vi "!GviewerMain.vi"() -> ()   [LabVIEW 2020, in "Sgraph_lib_V1.lvlib" / "Gviewer.lvclass"]
doc: "Main Graph Viewer.\nSeveral instances of this viewer can run simultaneously."
uses:
  Gviewer.lvclass
  controls/Typedef_Live.ctl
  Gserver/controls/Typedef_Gviewer-Query.ctl
  Gserver/controls/Typedef_QueryType.ctl
  controls/KeyPress.ctl
  <vilib>/event_ctls.llb/eventvkey.ctl
  Gviewer.lvclass/Gviewer.ctl
  FAMM/controls/FAMM_reply_datagram.ctl
  FAMM/controls/FAMM_reply_WAQdata.ctl
  FAMM/controls/FAMM_reply_EAQdata.ctl
  FAMM/controls/FAMM_reply_PAQdata.ctl
  controls/EditTagOneTag.ctl
  controls/Typedef_SelProperties.ctl
  controls/Typedef_LineType.ctl
  controls/Typedef_PresetSave.ctl
  controls/AutoScale.ctl
  controls/ToolBarAppearance.ctl
  controls/Typedef_Gserver-Replies.ctl
  controls/Typedef_ServerActions.ctl
  Common/controls/ToolTypeEnum.ctl
  controls/YgraphDef.ctl
  controls/MinMax.ctl
  Gserver/Gserver.lvclass
  FAMM/FAMM.lvclass
  Builds/Sgraph_lib_V1.lvlib
panel:
  out "TimeSpanText":string
  out "Key UP":T1 {"Time" format="%<%.3X>T"}
  out "Key DN":T1 {"Time" format="%<%.3X>T"}
  in  "StartupTagList":string[](array[string])
  in  "Gserver-Queue":refnum<queue>
  in  "GviewName":string="Gview-01"
  in  "Live":T3
  out "ToolBar":picture
  out "Graph":cluster{dbl[], "data":dbl[]}[](graph)
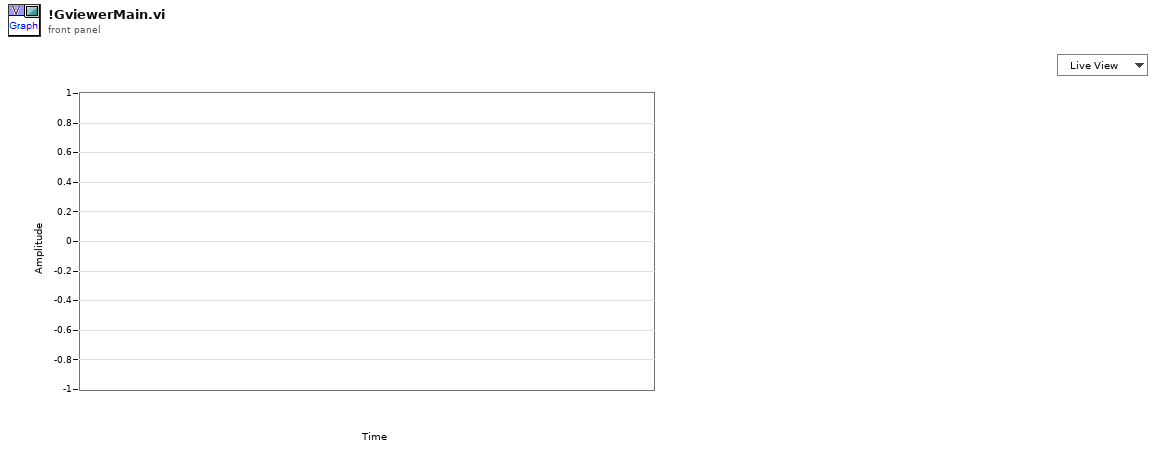
[diagram p1: front panel]
types:
  T1 = typedef "Sgraph_lib_V1.lvlib/Gviewer.lvclass/KeyPress.ctl" = cluster{"Char":i16, "VKey":T2, "Shift":bool, "Ctrl":bool, "Time":timestamp}
  T2 = typedef "eventvkey.ctl" = enum16{"ASCII", "Enter", "Return", "Shift", "Ctrl", "Alt", "Cmd", "Opt", "Caps", "NumLock", "Clear", "Break", "Up", "Down", "Left", "Right", "Insert", "Delete", "Home", "End", "PageUp", "PageDown", "Escape", "Help", "Pause", "ScrollLock", "F1", "F2", "F3", "F4", "F5", "F6", "F7", "F8", "F9", "F10", "F11", "F12", "F13", "F14", "F15", "F16", "F17", "F18", "F19", "F20", "F21", "F22", "F23", "F24", "Play", "VolumeUp", "VolumeDown", "Mute", "Two Byte Char"}
  T3 = typedef "Sgraph_lib_V1.lvlib/Gviewer.lvclass/Typedef_Live.ctl" = enum16{"Live View", "Freeze"}
  T4 = typedef "Sgraph_lib_V1.lvlib/FAMM.lvclass/FAMM_reply_datagram.ctl" = cluster{"GraphName":string, "Time-Start":timestamp, "Time-End":timestamp, "TimeSpan":dbl, "Live":T3, "WAQ_section":T5, "EAQ_section":T6, "PAQ_section":T7, "Layer":i32}
  T5 = typedef "Sgraph_lib_V1.lvlib/FAMM.lvclass/FAMM_reply_WAQdata.ctl" = cluster{"Boolean":bool}
  T6 = typedef "Sgraph_lib_V1.lvlib/FAMM.lvclass/FAMM_reply_EAQdata.ctl" = cluster{"Boolean":bool}
  T7 = typedef "Sgraph_lib_V1.lvlib/FAMM.lvclass/FAMM_reply_PAQdata.ctl" = cluster{"Tags":string[], "time stamp":timestamp[], "DataSection":cluster{"data":dbl[], "max":dbl[], "min":dbl[], "Status":u32[]}[]}
  T8 = typedef "Sgraph_lib_V1.lvlib/Gviewer.lvclass/EditTagOneTag.ctl" = cluster{"TAG":string, "min":dbl, "max":dbl, "Color":u32}
  T9 = typedef "Sgraph_lib_V1.lvlib/Gviewer.lvclass/Typedef_LineType.ctl" = enum16{"num_bare", "num_MinMax_Area", "num_MinMax_Lines", "num_MinMax_Forfor", "num_Max_Area", "num_Max_Line", "num_Max_Forfor", "num_Min_Area", "num_Min_Line", "num_Min_Fosfor", "Boolean_Line_01", "Boolean_Area_01", "Boolean_Fosfor_01", "Boolean_Line_TF", "Boolean_Area_TF", "Boolean_Fosfor_TF", "Boolean_OnOff_Line", "Boolean_OnOff_Area", "Boolean_OnOff_Fosfor", "Boolean_spare", "StringEvent_Line", "StringEvent_TimeLine"}
  T10 = typedef "Sgraph_lib_V1.lvlib/Gviewer.lvclass/Typedef_SelProperties.ctl" = cluster{"Color":u32, "LineType":T9, "max":dbl, "min":dbl}
  T11 = cluster{"EditTagsOpen":bool, "ExitRef":refnum<vi>}
  T12 = typedef "Sgraph_lib_V1.lvlib/Gviewer.lvclass/Typedef_PresetSave.ctl" = cluster{"Save time?":bool, "Presets":T8[], "PresetFilePath":path}
  T13 = typedef "Sgraph_lib_V1.lvlib/Gviewer.lvclass/AutoScale.ctl" = enum16{"FitEqual", "FitMax", "StackEqual", "StackMax", "StackPerType"}
  T14 = typedef "Sgraph_lib_V1.lvlib/Gserver.lvclass/Typedef_QueryType.ctl" = enum16{"Subscribe", "DataRequest", "RequestAllTags", "RequestIniPath", "FAMMstarted", "SetClientOptions", "GviewerUpdate", "OpenNewGraph", "CloseClient", "CloseAllClients", "Close Gserver", "OpenMemoryMap", "MeMapDataRequest", "MeMapDataResponse", "OpenDBeditor", "CheckDBeditorRunning", "StoppedDBeditor", "SaveDB_TAGpropRecord", "ConfirmDB_TAGpropSave"}
  T15 = typedef "Sgraph_lib_V1.lvlib/Gviewer.lvclass/ToolBarAppearance.ctl" = enum16{"Bare", "Native", "Gradient"}
  T16 = typedef "Sgraph_lib_V1.lvlib/Gviewer.lvclass/Typedef_ServerActions.ctl" = enum16{"GraphUpdate", "SendAllTags", "SendIniPath", "SetGeneralOptions", "EditTagsOpen", "EditTagsPresetSave", "EditTagsPresetLoad", "EditTagsClose", "NewTagSelection", "AutoScale", "DBeditStatus", "DBsaveConfirm", "ExitGraph"}
  T17 = typedef "Typedef_Gserver-Replies.ctl" = cluster{"ServerActions":T16, "data":variant, "Source":string, "Time Stamp":timestamp}
  T18 = typedef "Sgraph_lib_V1.lvlib/ToolTypeEnum.ctl" = enum16{"00_Esc button", "01_Undo", "02_HelpButton", "03_CursorViewButton", "04_AutoScale_Fit", "05_AutoScale_Stacked", "06_ZoomWindowStart", "07_ZoomTimeStart", "08_ZoomAmplitudeStart", "09", "10", "11", "12", "13", "14", "15", "16", "17", "18", "19", "20_VerticalScroll", "21_VerticalMove", "22_TimeScroll", "23_TimeMove", "24", "25", "26_ZoomWindowSize", "27_ZoomTimeWindowSize", "28_ZoomAmplitudeWindowSize", "29", "30_LegendMovePoint", "31_LegendMoveDrag", "32", "33", "34", "35", "36", "37", "38", "39", "40_AddYscalePoint", "41_AddYscalePlace", "42_AddYscaleMovePoint", "43_AddYscaleMoveDrag", "44_AddYscaleDeletePoint"}
  T19 = typedef "Sgraph_lib_V1.lvlib/Gviewer.lvclass/YgraphDef.ctl" = cluster{"Plot":i32, "X(%)":dbl}
  T20 = typedef "Sgraph_lib_V1.lvlib/Gviewer.lvclass/MinMax.ctl" = enum16{"On", "Off", "Focus"}
  T21 = typedef "Sgraph_lib_V1.lvlib/Gviewer.lvclass/SettingsGeneral.ctl" = cluster{"MenuBar_active":bool, "ContextMenu_active":bool}
  T22 = typedef "LVPositionTypeDef.ctl" = cluster{"Left":i32, "Top":i32}
  T23 = typedef "LVPoint32TypeDef.ctl" = cluster{"Horizontal":i32, "Vertical":i32}
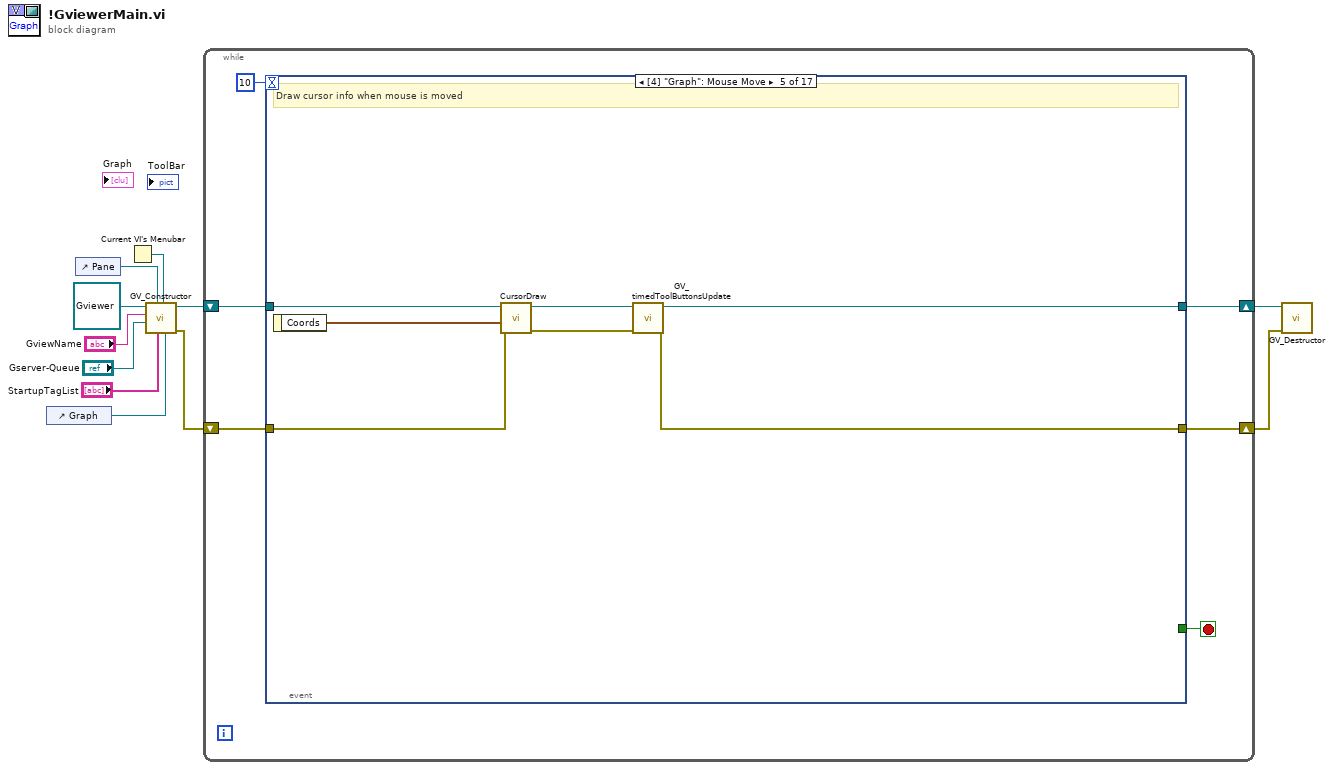
[diagram p0: block diagram]
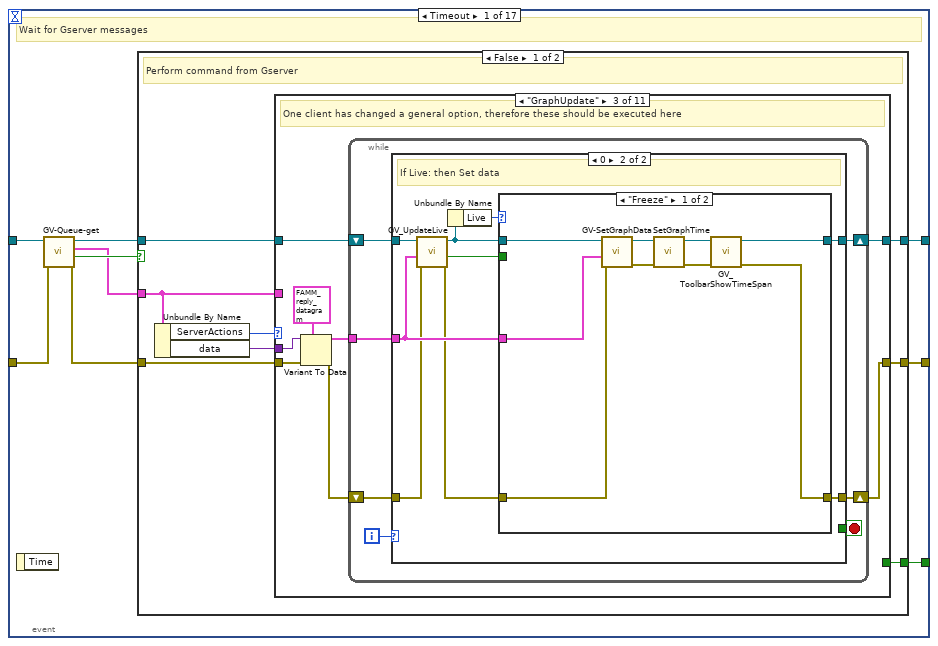
[diagram p2: hidden frame]
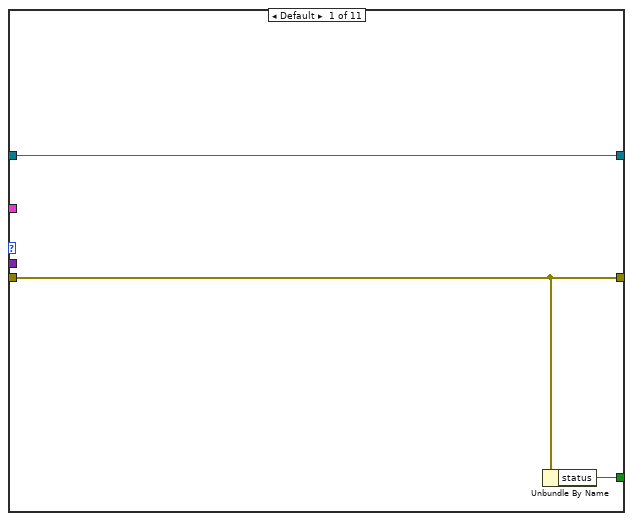
[diagram p3: hidden frame]
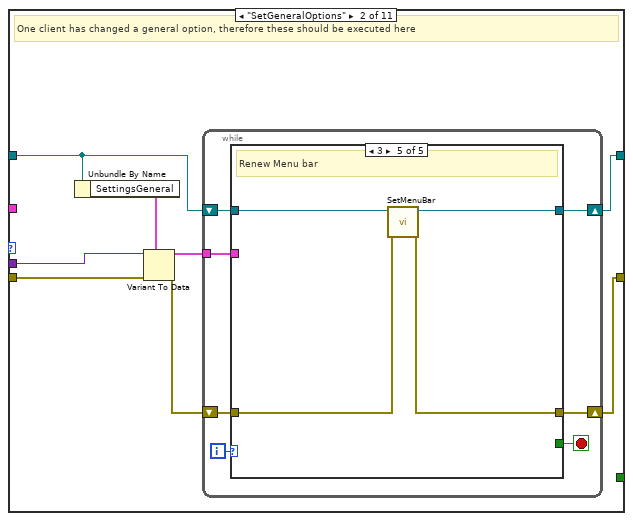
[diagram p4: hidden frame]
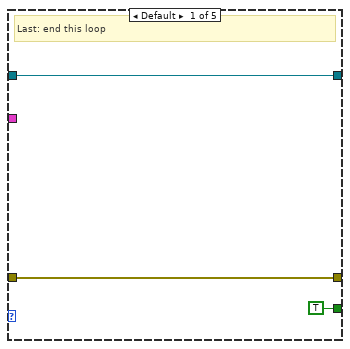
[diagram p5: hidden frame]
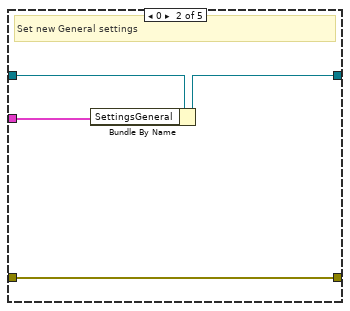
[diagram p6: hidden frame]
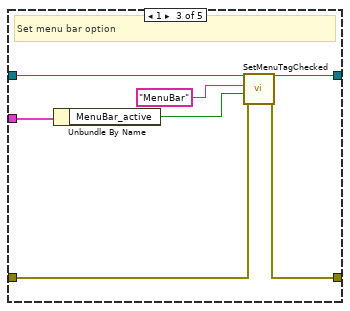
[diagram p7: hidden frame]
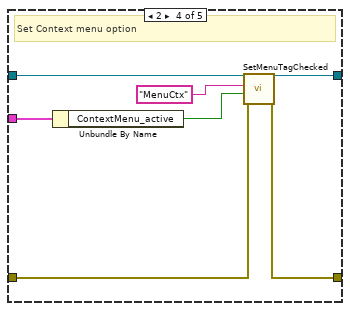
[diagram p8: hidden frame]
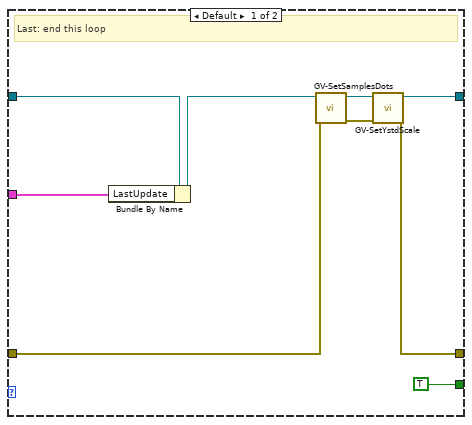
[diagram p9: hidden frame]
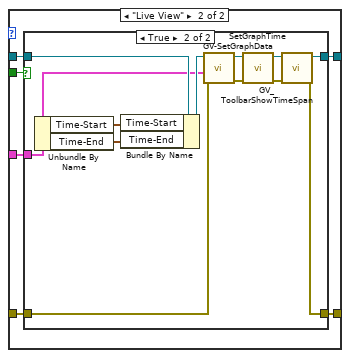
[diagram p10: hidden frame]
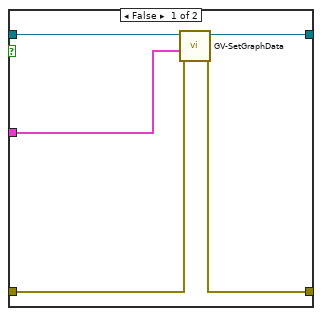
[diagram p11: hidden frame]
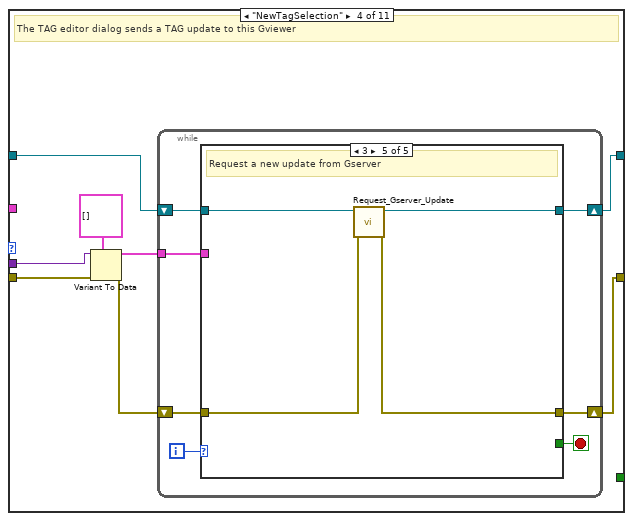
[diagram p12: hidden frame]
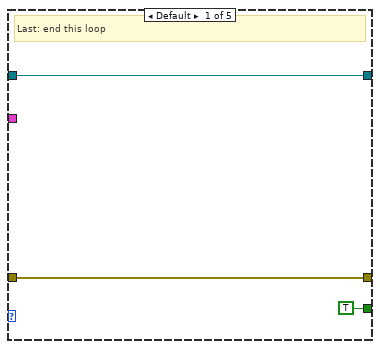
[diagram p13: hidden frame]
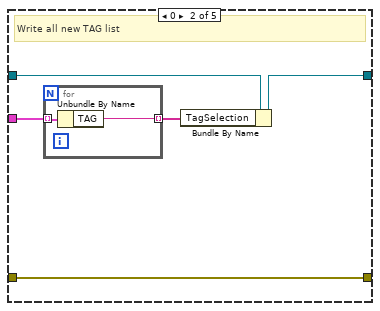
[diagram p14: hidden frame]
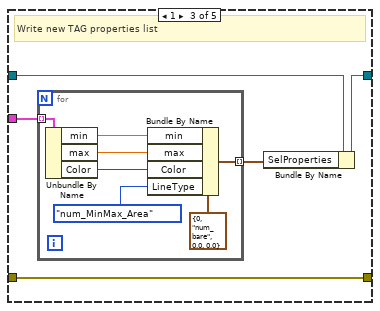
[diagram p15: hidden frame]
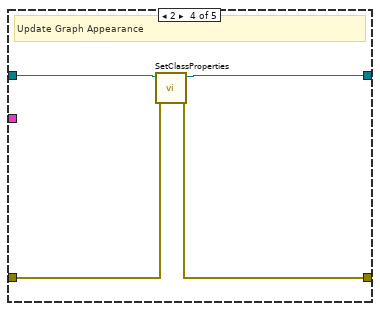
[diagram p16: hidden frame]
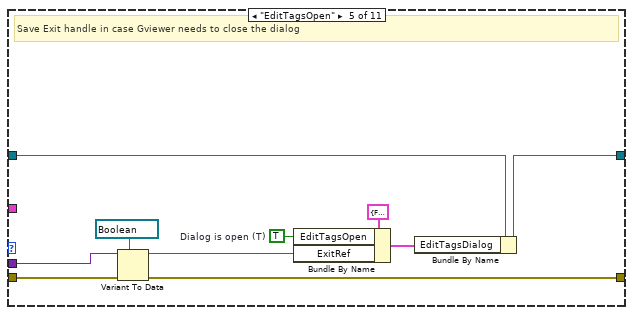
[diagram p17: hidden frame]
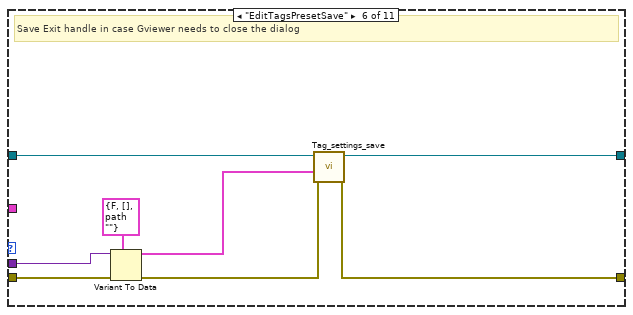
[diagram p18: hidden frame]
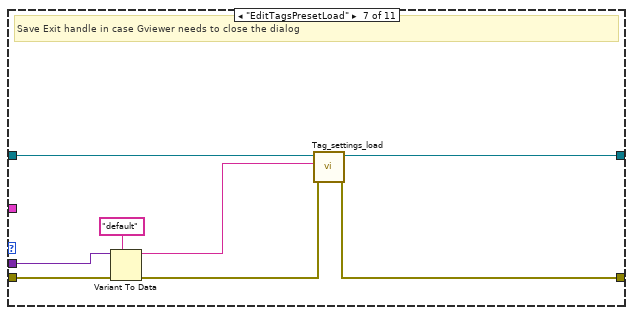
[diagram p19: hidden frame]
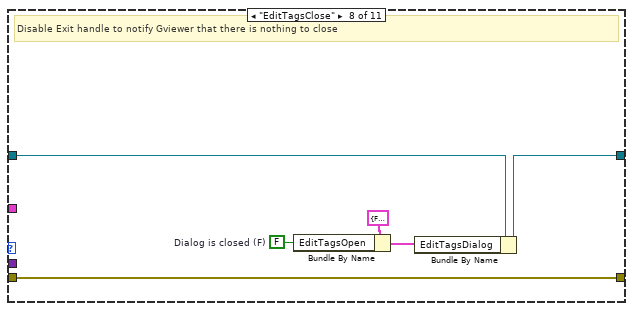
[diagram p20: hidden frame]
diagram:
  n1 = control-ref of="Graph"() -> (w2:refnum<vi>)
  n2 = control-ref of="Pane"() -> (w8:refnum<vi>)
  n3 = Current VI's Menubar() -> (w3:refnum<k9>)
  n4 = call "GV_Constructor.vi"("Graph-ref"=w2, "menu reference"=w3, "StartupTagList"="StartupTagList", "Pane"=w8, "Gserver-Queue"="Gserver-Queue", "GviewName"="GviewName", "Gviewer in"=refnum<class "Gviewer.lvclass"> refnum) -> ("error out"=w4:errorcluster, "Gviewer out"=w11:refnum<class "Gviewer.lvclass">)  [unwired: 3 in]
  n5 = while {
    shift-right: [w15] -> w1
    shift-left: w11 -> [w16]
    shift-right: [w13] -> w10
    shift-left: w4 -> [w14]
    stop <- w12 stop-if-true
    n6 = event shown="[4] \"Graph\": Mouse Move" {
      selector: _ -> [_ _ _ _ _ _ _ _ _ _ _ _ _ _ _ _ _]
      dyn-events: _ -> [_ _ _ _ _ _ _ _ _ _ _ _ _ _ _ _ _]
      timeout: 10 -> [_ _ _ _ _ _ _ _ _ _ _ _ _ _ _ _ _]
      tunnel: w16 -> [w19 w261 w276 w878 w889 w899 w904 w911 w945 w957 w996 w1018 w1026 w1035 w1104 w1116 w1120]
      tunnel: [w25 w255 w274 w871 w887 w894 w905 w909 w946 w952 w990 w1019 w1022 w1028 w1101 w1109 w1119] -> w15
      tunnel: w14 -> [w21 w259 w275 w877 w893 w897 w902 w910 w943 w956 w995 w1016 w1025 w1033 w1106 w1107 w1117]
      tunnel: [w26 w257 w273 w870 w890 w898 w903 w908 w944 w950 w987 w1017 w1020 w1030 w1105 w1108 w1117] -> w13
      tunnel: [w24 _ _ _ _ _ _ _ _ _ _ _ _ _ _ _ _] -> w12
      event Timeout {
        # "Wait for Gserver messages"
        n7 = event-data() -> ()  [unwired: 1 in, 1 out]
        n8 = call "GV-Queue-get.vi"("error in (no error)"=w21, "Gviewer in"=w19) -> ("error out"=w20:errorcluster, "Time-out"=w23:bool, "Query"=w22:T17, "Gviewer out"=w18:refnum<class "Gviewer.lvclass">)  [unwired: 6 in]
        n9 = case shown="False" w23 {
          tunnel: w22 -> [w27 _]
          tunnel: w18 -> [w33 w249]
          tunnel: w20 -> [w32 w251]
          tunnel: [w31 w252] -> w26
          tunnel: [w30 w250] -> w25
          tunnel: [w29 w253] -> w24
          frame False {
            # "Perform command from Gserver"
            n10 = Unbundle By Name(w27) -> ("ServerActions"=w34:T16, "data"=w28:variant)
            n11 = case shown="\"GraphUpdate\"" w34 {
              tunnel: w33 -> [w37 w39 w80 w145 w188 w201 w211 w218 w224 w235 w241]
              tunnel: w32 -> [w35 w44 w84 w149 w194 w204 w212 w214 w226 w229 w238]
              tunnel: [w35 w40 w81 w146 w195 w198 w208 w214 w221 w233 w236] -> w31
              tunnel: [w37 w42 w83 w148 w193 w202 w210 w219 w225 w234 w241] -> w30
              tunnel: [w36 _ _ _ _ _ _ _ _ _ TRUE] -> w29
              tunnel: w27 -> [_ _ _ _ _ _ _ _ _ _ _]
              tunnel: w28 -> [_ w45 w85 w150 w197 w205 w213 _ w227 w232 _]
              frame Default {
                n12 = Unbundle By Name(w35) -> ("status"=w36:bool)
              }
              frame "SetGeneralOptions" {
                # "One client has changed a general option, therefore these should be executed here"
                n13 = Unbundle By Name(w39) -> ("SettingsGeneral"=w43:T21)
                n14 = Variant To Data(error in=w44, type=w43, Variant=w45) -> (data=w38:T21, error out=w41:errorcluster)
                n15 = while {
                  shift-right: [w47] -> w42
                  shift-left: w39 -> [w50]
                  shift-right: [w46] -> w40
                  shift-left: w41 -> [w49]
                  tunnel: w38 -> [w48]
                  i -> [w52]
                  stop <- w51 stop-if-true
                  n16 = case shown="3" w52 {
                    tunnel: [TRUE _ _ _ _] -> w51
                    tunnel: w50 -> [w53 w59 w61 w72 w77]
                    tunnel: w49 -> [w54 w56 w63 w68 w75]
                    tunnel: w48 -> [_ w58 w60 w70 _]
                    tunnel: [w53 w57 w65 w71 w76] -> w47
                    tunnel: [w54 w56 w62 w67 w74] -> w46
                    frame Default {
                      # "Last: end this loop"
                    }
                    frame 0 {
                      # "Set new General settings"
                      n17 = Bundle By Name(cluster=w59, "SettingsGeneral"=w58) -> (w57:refnum<class "Gviewer.lvclass">)
                    }
                    frame 1 {
                      # "Set menu bar option"
                      n18 = Unbundle By Name(w60) -> ("MenuBar_active"=w64:bool)
                      n19 = call "SetMenuTagChecked.vi"("error in (no error)"=w63, "Checked"=w64, "TAG"="MenuBar", "Gviewer in"=w61) -> ("error out"=w62:errorcluster, "Gviewer out"=w65:refnum<class "Gviewer.lvclass">)  [unwired: 6 in]
                    }
                    frame 2 {
                      # "Set Context menu option"
                      n20 = Unbundle By Name(w70) -> ("ContextMenu_active"=w69:bool)
                      n21 = call "SetMenuTagChecked.vi"("error in (no error)"=w68, "Checked"=w69, "TAG"="MenuCtx", "Gviewer in"=w72) -> ("error out"=w67:errorcluster, "Gviewer out"=w71:refnum<class "Gviewer.lvclass">)  [unwired: 6 in]
                    }
                    frame 3 {
                      # "Renew Menu bar"
                      n22 = call "SetMenuBar.vi"("error in (no error)"=w75, "Gviewer in"=w77) -> ("error out"=w74:errorcluster, "Gviewer out"=w76:refnum<class "Gviewer.lvclass">)  [unwired: 8 in]
                    }
                  }
                }
              }
              frame "GraphUpdate" {
                # "One client has changed a general option, therefore these should be executed here"
                n23 = Variant To Data(error in=w84, type=T4 {"GraphName"="", "Time-Start"=timestamp(0 s since 1904-01-01), "Time-End"=timestamp(0 s since 1904-01-01), "TimeSpan"=0.0, "Live"=enum."Live View", "WAQ_section"={"Boolean"=FALSE}, "EAQ_section"={"Boolean"=FALSE}, "PAQ_section"={"Tags"=[], "time stamp"=[], "DataSection"=[]}, "Layer"=0} ("GviewerUpdate"), Variant=w85) -> (data=w79:T4, error out=w82:errorcluster)
                n24 = while {
                  shift-right: [w87] -> w83
                  shift-left: w80 -> [w90]
                  shift-right: [w86] -> w81
                  shift-left: w82 -> [w89]
                  tunnel: w79 -> [w88]
                  i -> [w92]
                  stop <- w91 stop-if-true
                  n25 = case shown="0" w92 {
                    tunnel: [TRUE _] -> w91
                    tunnel: w90 -> [w98 w108]
                    tunnel: w89 -> [w94 w105]
                    tunnel: w88 -> [w93 w107]
                    tunnel: [w99 w110] -> w87
                    tunnel: [w100 w109] -> w86
                    frame Default {
                      # "Last: end this loop"
                      n26 = Bundle By Name(cluster=w98, "LastUpdate"=w93) -> (w97:refnum<class "Gviewer.lvclass">)
                      n27 = call "GV-SetSamplesDots.vi"("error in (no error)"=w94, "Gviewer in"=w97) -> ("error out"=w95:errorcluster, "Gviewer out"=w96:refnum<class "Gviewer.lvclass">)  [unwired: 8 in]
                      n28 = call "GV-SetYstdScale.vi"("error in (no error)"=w95, "Gviewer in"=w96) -> ("error out"=w100:errorcluster, "Gviewer out"=w99:refnum<class "Gviewer.lvclass">)  [unwired: 8 in]
                    }
                    frame 0 {
                      # "If Live: then Set data"
                      n29 = call "GV_UpdateLive.vi"("error in (no error)"=w105, "GviewerUpdate"=w107, "Gviewer in"=w108) -> ("error out"=w106:errorcluster, "RollTime?"=w102:bool, "Gviewer out"=w104:refnum<class "Gviewer.lvclass">)  [unwired: 6 in]
                      n30 = Unbundle By Name(w104) -> ("Live"=w103:T3)
                      n31 = case shown="\"Freeze\"" w103 {
                        tunnel: w104 -> [w119 w125]
                        tunnel: [w113 w124] -> w110
                        tunnel: w106 -> [w118 w123]
                        tunnel: [w111 w122] -> w109
                        tunnel: w107 -> [w117 w121]
                        tunnel: w102 -> [_ w120]
                        frame "Freeze" {
                          n32 = call "GV-SetGraphData.vi"("error in (no error)"=w118, "GviewerUpdate"=w117, "Gviewer in"=w119) -> ("error out"=w115:errorcluster, "Gviewer out"=w116:refnum<class "Gviewer.lvclass">)  [unwired: 7 in]
                          n33 = call "SetGraphTime.vi"("error in (no error)"=w115, "Gviewer in"=w116) -> ("error out"=w112:errorcluster, "Gviewer out"=w114:refnum<class "Gviewer.lvclass">)  [unwired: 8 in]
                          n34 = call "GV_ToolbarShowTimeSpan.vi"("error in (no error)"=w112, "Gviewer in"=w114) -> ("error out"=w111:errorcluster, "Gviewer out"=w113:refnum<class "Gviewer.lvclass">)  [unwired: 7 in, 1 out]
                        }
                        frame "Live View" {
                          n35 = case shown="True" w120 {
                            tunnel: w125 -> [w130 w138]
                            tunnel: [w129 w132] -> w124
                            tunnel: w123 -> [w128 w142]
                            tunnel: [w127 w131] -> w122
                            tunnel: w121 -> [w126 w137]
                            frame False {
                              n36 = call "GV-SetGraphData.vi"("error in (no error)"=w128, "GviewerUpdate"=w126, "Gviewer in"=w130) -> ("error out"=w127:errorcluster, "Gviewer out"=w129:refnum<class "Gviewer.lvclass">)  [unwired: 7 in]
                            }
                            frame True {
                              n37 = Unbundle By Name(w137) -> ("Time-Start"=w135:timestamp, "Time-End"=w136:timestamp)
                              n38 = Bundle By Name(cluster=w138, "Time-Start"=w135, "Time-End"=w136) -> (w139:refnum<class "Gviewer.lvclass">)
                              n39 = call "GV-SetGraphData.vi"("error in (no error)"=w142, "GviewerUpdate"=w137, "Gviewer in"=w139) -> ("error out"=w140:errorcluster, "Gviewer out"=w141:refnum<class "Gviewer.lvclass">)  [unwired: 7 in]
                              n40 = call "SetGraphTime.vi"("error in (no error)"=w140, "Gviewer in"=w141) -> ("error out"=w133:errorcluster, "Gviewer out"=w134:refnum<class "Gviewer.lvclass">)  [unwired: 8 in]
                              n41 = call "GV_ToolbarShowTimeSpan.vi"("error in (no error)"=w133, "Gviewer in"=w134) -> ("error out"=w131:errorcluster, "Gviewer out"=w132:refnum<class "Gviewer.lvclass">)  [unwired: 7 in, 1 out]
                            }
                          }
                        }
                      }
                    }
                  }
                }
              }
              frame "NewTagSelection" {
                # "The TAG editor dialog sends a TAG update to this Gviewer"
                n42 = Variant To Data(error in=w149, type=T8[] [] ("Presets"), Variant=w150) -> (data=w144:T8[], error out=w147:errorcluster)
                n43 = while {
                  shift-right: [w152] -> w148
                  shift-left: w145 -> [w155]
                  shift-right: [w151] -> w146
                  shift-left: w147 -> [w154]
                  tunnel: w144 -> [w153]
                  i -> [w157]
                  stop <- w156 stop-if-true
                  n44 = case shown="3" w157 {
                    tunnel: [TRUE _ _ _ _] -> w156
                    tunnel: w155 -> [w158 w164 w170 w183 w186]
                    tunnel: w154 -> [w159 w161 w172 w181 w184]
                    tunnel: w153 -> [_ w165 w169 _ _]
                    tunnel: [w158 w162 w171 w180 w187] -> w152
                    tunnel: [w159 w161 w172 w182 w185] -> w151
                    frame Default {
                      # "Last: end this loop"
                    }
                    frame 0 {
                      # "Write all new TAG list"
                      n45 = for {
                        tunnel: w165 -> [w167] mode=indexing
                        tunnel: [w166] -> w163 mode=indexing
                        n46 = Unbundle By Name(w167) -> ("TAG"=w166:string)
                      }
                      n47 = Bundle By Name(cluster=w164, "TagSelection"=w163) -> (w162:refnum<class "Gviewer.lvclass">)
                    }
                    frame 1 {
                      # "Write new TAG properties list"
                      n48 = for {
                        tunnel: w169 -> [w179] mode=indexing
                        tunnel: [w173] -> w168 mode=indexing
                        n49 = Unbundle By Name(w179) -> ("min"=w177:dbl, "max"=w176:dbl, "Color"=w175:u32)
                        n50 = Bundle By Name(cluster=T10 {"Color"=0, "LineType"=enum."num_bare", "max"=0.0, "min"=0.0} ("SelProperties"), "min"=w177, "max"=w176, "Color"=w175, "LineType"=Typedef_LineType."num_MinMax_Area") -> (w173:T10)
                      }
                      n51 = Bundle By Name(cluster=w170, "SelProperties"=w168) -> (w171:refnum<class "Gviewer.lvclass">)
                    }
                    frame 2 {
                      # "Update Graph Appearance"
                      n52 = call "SetClassProperties.vi"("error in (no error)"=w181, "Gviewer in"=w183) -> ("error out"=w182:errorcluster, "Gviewer out"=w180:refnum<class "Gviewer.lvclass">)  [unwired: 8 in]
                    }
                    frame 3 {
                      # "Request a new update from Gserver"
                      n53 = call "Request_Gserver_Update.vi"("error in (no error)"=w184, "Gviewer in"=w186) -> ("error out"=w185:errorcluster, "Gviewer out"=w187:refnum<class "Gviewer.lvclass">)  [unwired: 8 in]
                    }
                  }
                }
              }
              frame "EditTagsOpen" {
                w191 = TRUE  # Dialog is open (T)
                # "Save Exit handle in case Gviewer needs to close the dialog"
                n54 = Variant To Data(error in=w194, type=refnum<vi> refnum ("Exit_event"), Variant=w197) -> (data=w190:refnum<vi>, error out=w195:errorcluster)
                n55 = Bundle By Name(cluster=T11 {"EditTagsOpen"=FALSE, "ExitRef"=refnum} ("EditTagsDialog"), "EditTagsOpen"=w191, "ExitRef"=w190) -> (w189:T11)
                n56 = Bundle By Name(cluster=w188, "EditTagsDialog"=w189) -> (w193:refnum<class "Gviewer.lvclass">)
              }
              frame "EditTagsPresetSave" {
                # "Save Exit handle in case Gviewer needs to close the dialog"
                n57 = Variant To Data(error in=w204, type=T12 {"Save time?"=FALSE, "Presets"=[], "PresetFilePath"=path ""} ("PresetSave"), Variant=w205) -> (data=w200:T12, error out=w199:errorcluster)
                n58 = call "Tag_settings_save.vi"("error in (no error)"=w199, "PresetSave"=w200, "Gviewer in"=w201) -> ("error out"=w198:errorcluster, "Gviewer out"=w202:refnum<class "Gviewer.lvclass">)  [unwired: 7 in]
              }
              frame "EditTagsPresetLoad" {
                # "Save Exit handle in case Gviewer needs to close the dialog"
                n59 = Variant To Data(error in=w212, type="default", Variant=w213) -> (data=w206:string, error out=w209:errorcluster)
                n60 = call "Tag_settings_load.vi"("error in (no error)"=w209, "PresetName"=w206, "Gviewer in"=w211) -> ("error out"=w208:errorcluster, "Gviewer out"=w210:refnum<class "Gviewer.lvclass">)  [unwired: 7 in]
              }
              frame "EditTagsClose" {
                w216 = FALSE  # Dialog is closed (F)
                # "Disable Exit handle to notify Gviewer that there is nothing to close"
                n61 = Bundle By Name(cluster=T11 {"EditTagsOpen"=FALSE, "ExitRef"=refnum} ("EditTagsDialog"), "EditTagsOpen"=w216) -> (w215:T11)
                n62 = Bundle By Name(cluster=w218, "EditTagsDialog"=w215) -> (w219:refnum<class "Gviewer.lvclass">)
              }
              frame "AutoScale" {
                # "Perform Autoscale on Graph"
                n63 = Variant To Data(error in=w226, type=AutoScale."FitEqual" ("AutoScale"), Variant=w227) -> (data=w223:T13, error out=w222:errorcluster)
                n64 = call "GV_AutoScale.vi"("error in (no error)"=w222, "AutoScale"=w223, "Gviewer in"=w224) -> ("error out"=w221:errorcluster, "Gviewer out"=w225:refnum<class "Gviewer.lvclass">)  [unwired: 7 in]
              }
              frame "DBeditStatus" {
                w231 = TRUE  # Started?
                # "Receive the DBedit status from Gserver"
                n65 = Variant To Data(error in=w229, type=w231, Variant=w232) -> (data=w228:bool, error out=w230:errorcluster)
                n66 = call "GV_DBeditReply.vi"("error in (no error)"=w230, "Started?"=w228, "Gviewer in"=w235) -> ("error out"=w233:errorcluster, "Gviewer out"=w234:refnum<class "Gviewer.lvclass">)  [unwired: 7 in]
              }
              frame "ExitGraph" {
                # "Exit this Graph application (shutdown asked by Gserver)"
                n67 = Unbundle By Name(w241) -> ("EditTagsDialog"=w240:T11)
                n68 = Unbundle By Name(w240) -> ("ExitRef"=w237:refnum<vi>, "EditTagsOpen"=w239:bool)
                n69 = case "Close TAG edit dialog" shown="True" w239 {
                  selector: w239 -> [_ w245]
                  tunnel: w238 -> [w243 w247]
                  tunnel: w237 -> [_ w248]
                  tunnel: [w243 w246] -> w236
                  frame False {
                  }
                  frame True {
                    n70 = To Variant(anything=w245) -> (Variant=w244:variant)
                    n71 = property class="Bool"(reference=w248, error in=w247, "Val(Sgnl)"=w244) -> (error out=w246:errorcluster)  [unwired: 1 out]
                  }
                }
              }
            }
          }
          frame True {
            # "Receiving Queue time-out"
            n72 = call "GV-EventsProcessing.vi"("error in (no error)"=w251, "Gviewer in"=w249) -> ("error out"=w252:errorcluster, "Gviewer out"=w250:refnum<class "Gviewer.lvclass">)  [unwired: 8 in]
            n73 = Unbundle By Name(w252) -> ("status"=w253:bool)
          }
        }
      }
      event Shortcut Menu Activation? {
        # "Right mouse click menu selection"
        n74 = event-data() -> ("MenuRef"=w260:refnum<k9>)  [unwired: 1 in]
        n75 = Unbundle By Name(w261) -> ("Context_set"=w262:bool)
        n76 = case shown="False" w262 {
          selector: w262 -> [w268 _]
          tunnel: w261 -> [w265 w269]
          tunnel: w260 -> [w266 w271]
          tunnel: w259 -> [w263 w272]
          tunnel: [w263 w272] -> w256
          tunnel: [w264 w270] -> w258
          frame False {
            n77 = Not(x=w268) -> (.not. x?=w267:bool)
            n78 = Bundle By Name(cluster=w265, "Context_set"=w267, "Context-ref"=w266) -> (w264:refnum<class "Gviewer.lvclass">)
          }
          frame True {
            n79 = Bundle By Name(cluster=w269, "Context-ref"=w271) -> (w270:refnum<class "Gviewer.lvclass">)
          }
        }
        n80 = call "SetContextMenu.vi"("error in (no error)"=w256, "Gviewer in"=w258) -> ("error out"=w257:errorcluster, "Gviewer out"=w255:refnum<class "Gviewer.lvclass">)  [unwired: 8 in]
        n81 = event-data("Discard?"=FALSE) -> ()  [unwired: 1 in, 1 out]
      }
      event Menu Selection (User); Shortcut Menu Selection (User) {
        # "Menu bar action"
        n82 = event-data() -> ("ItemTag"=w277:string)  [unwired: 1 in]
        n83 = case shown="\"MinMaxFocus\", \"MinMaxOff\", \"MinMaxOn\"" w277 {
          selector: w277 -> [_ _ _ _ w328 _ w525 _ _ w590 _ _ _ _ w645 _ _ _ _ _ _ _ _ _ _ _ _ _ _ w854 w862]
          tunnel: w276 -> [w281 w286 w296 w310 w326 w508 w523 w534 w537 w585 w591 w599 w611 w631 w642 w646 w657 w666 w676 w691 w709 w727 w743 w760 w777 w795 w813 w832 w847 w848 w863]
          tunnel: w275 -> [w280 w285 w290 w309 w325 w505 w526 w532 w551 w581 w598 w606 w609 w624 w640 w651 w653 w662 w678 w693 w711 w729 w745 w762 w779 w797 w815 w833 w845 w852 w859]
          tunnel: [w282 w287 w292 w315 w323 w507 w528 w535 w537 w578 w592 w600 w612 w626 w639 w652 w661 w670 w687 w703 w721 w739 w755 w772 w789 w807 w825 w843 w846 w853 w863] -> w274
          tunnel: [w279 w284 w291 w313 w321 w506 w527 w533 w552 w575 w598 w606 w608 w625 w632 w650 w660 w669 w686 w702 w720 w738 w754 w771 w788 w806 w824 w842 w844 w851 w859] -> w273
          frame "Exit" {
            # "Send Exit command to Gserver (Gserver will then close this application)"
            n84 = call "SendDataToServer.vi"("error in (no error)"=w280, "Query_type"=Typedef_QueryType."CloseClient", "Gviewer in"=w281) -> ("error out"=w279:errorcluster, "Gviewer out"=w282:refnum<class "Gviewer.lvclass">)  [unwired: 7 in]
          }
          frame "ExitAll" {
            # "Send Exit command to Gserver (Gserver will then close this application)"
            n85 = call "SendDataToServer.vi"("error in (no error)"=w285, "Query_type"=Typedef_QueryType."CloseAllClients", "Gviewer in"=w286) -> ("error out"=w284:errorcluster, "Gviewer out"=w287:refnum<class "Gviewer.lvclass">)  [unwired: 7 in]
          }
          frame "MenuBar" {
            # "Options: Menu bar"
            n86 = Unbundle By Name(w296) -> ("SettingsGeneral"=w298:T21)
            n87 = Unbundle By Name(w298) -> ("MenuBar_active"=w299:bool, "ContextMenu_active"=w295:bool)
            n88 = case shown="True" w299 {
              selector: w299 -> [w302 w304]
              tunnel: [w301 w306] -> w297
              tunnel: w295 -> [w300 w305]
              tunnel: [w300 w303] -> w294
              frame False {
                n89 = Not(x=w302) -> (.not. x?=w301:bool)
              }
              frame True {
                # "Contect bar must be active\nif menu bar is set to OFF"
                n90 = Or(x=w304, y=w305) -> (x .or. y?=w303:bool)
                n91 = Not(x=w304) -> (.not. x?=w306:bool)
              }
            }
            n92 = Bundle By Name(cluster=w298, "MenuBar_active"=w297, "ContextMenu_active"=w294) -> (w288:T21)
            n93 = Bundle By Name(cluster=w296, "SettingsGeneral"=w288) -> (w293:refnum<class "Gviewer.lvclass">)
            n94 = call "SendDataToServer.vi"("error in (no error)"=w290, "data"=w288, "Query_type"=Typedef_QueryType."SetClientOptions", "Gviewer in"=w293) -> ("error out"=w291:errorcluster, "Gviewer out"=w292:refnum<class "Gviewer.lvclass">)  [unwired: 6 in]
          }
          frame "Legend" {
            # "Options: Legend on/off"
            n95 = call "GV_LegendVisible.vi"("error in (no error)"=w309, "Gviewer in"=w310) -> ("error out"=w307:errorcluster, "Visible?"=w308:bool, "Gviewer out"=w311:refnum<class "Gviewer.lvclass">)  [unwired: 7 in]
            n96 = call "SetMenuTagChecked.vi"("error in (no error)"=w307, "Checked"=w308, "TAG"="Legend", "Gviewer in"=w311) -> ("error out"=w314:errorcluster, "Gviewer out"=w316:refnum<class "Gviewer.lvclass">)  [unwired: 6 in]
            n97 = call "SetMenuBar.vi"("error in (no error)"=w314, "Gviewer in"=w316) -> ("error out"=w313:errorcluster, "Gviewer out"=w315:refnum<class "Gviewer.lvclass">)  [unwired: 8 in]
          }
          frame "T_000".."T_zzz" {
            # "Set Timeline"
            n98 = Get Date/Time In Seconds() -> (seconds since 1Jan1904=w327:timestamp)
            n99 = case shown="\"T_8hr\"" w328 {
              tunnel: w327 -> [_ _ _ _ _ _ _ w384 w397 w410 w423 _ _ _ _ _ _ _ _ _]
              tunnel: w326 -> [w330 w332 w340 w348 w356 w364 w372 w390 w403 w416 w429 w432 w440 w448 w456 w464 w472 w480 w488 w496]
              tunnel: w325 -> [w329 w338 w346 w354 w362 w370 w378 w387 w400 w413 w426 w438 w446 w454 w462 w470 w478 w486 w494 w502]
              tunnel: [w330 w334 w342 w350 w358 w366 w374 w391 w404 w417 w430 w434 w442 w450 w458 w466 w474 w482 w490 w498] -> w320
              tunnel: [w329 w338 w346 w354 w362 w370 w378 w385 w398 w411 w424 w438 w446 w454 w462 w470 w478 w486 w494 w502] -> w318
              frame Default {
                # "Not familiar.. Don't change"
              }
              frame "T_30sec" {
                w333 = 30.0  # 30 seconds
                # "Time span selected: 30 seconds"
                n100 = Unbundle By Name(w332) -> ("Time-End"=w331:timestamp)
                n101 = To Double Precision Float(number=w331) -> (double precision float=w337:dbl)
                n102 = Subtract(x=w337, y=w333) -> (x-y=w336:dbl)
                n103 = To Time Stamp(1:w336) -> (0:w335:timestamp)
                n104 = Bundle By Name(cluster=w332, "Time-Start"=w335, "TimeSpan(sec)"=w333) -> (w334:refnum<class "Gviewer.lvclass">)
              }
              frame "T_2min" {
                w341 = 120.0  # 2 minutes
                # "Time span selected: 2 minutes"
                n105 = Unbundle By Name(w340) -> ("Time-End"=w339:timestamp)
                n106 = To Double Precision Float(number=w339) -> (double precision float=w345:dbl)
                n107 = Subtract(x=w345, y=w341) -> (x-y=w344:dbl)
                n108 = To Time Stamp(1:w344) -> (0:w343:timestamp)
                n109 = Bundle By Name(cluster=w340, "Time-Start"=w343, "TimeSpan(sec)"=w341) -> (w342:refnum<class "Gviewer.lvclass">)
              }
              frame "T_10min" {
                w349 = 600.0  # 10 minutes
                # "Time span selected: 10 minutes"
                n110 = Unbundle By Name(w348) -> ("Time-End"=w347:timestamp)
                n111 = To Double Precision Float(number=w347) -> (double precision float=w353:dbl)
                n112 = Subtract(x=w353, y=w349) -> (x-y=w352:dbl)
                n113 = To Time Stamp(1:w352) -> (0:w351:timestamp)
                n114 = Bundle By Name(cluster=w348, "Time-Start"=w351, "TimeSpan(sec)"=w349) -> (w350:refnum<class "Gviewer.lvclass">)
              }
              frame "T_1hr" {
                w357 = 3600.0  # 60 minutes
                # "Time span selected: 1 hour"
                n115 = Unbundle By Name(w356) -> ("Time-End"=w355:timestamp)
                n116 = To Double Precision Float(number=w355) -> (double precision float=w361:dbl)
                n117 = Subtract(x=w361, y=w357) -> (x-y=w360:dbl)
                n118 = To Time Stamp(1:w360) -> (0:w359:timestamp)
                n119 = Bundle By Name(cluster=w356, "Time-Start"=w359, "TimeSpan(sec)"=w357) -> (w358:refnum<class "Gviewer.lvclass">)
              }
              frame "T_4hr" {
                w365 = 14400.0  # 4 hours
                # "Time span selected: 4 hours"
                n120 = Unbundle By Name(w364) -> ("Time-End"=w363:timestamp)
                n121 = To Double Precision Float(number=w363) -> (double precision float=w369:dbl)
                n122 = Subtract(x=w369, y=w365) -> (x-y=w368:dbl)
                n123 = To Time Stamp(1:w368) -> (0:w367:timestamp)
                n124 = Bundle By Name(cluster=w364, "Time-Start"=w367, "TimeSpan(sec)"=w365) -> (w366:refnum<class "Gviewer.lvclass">)
              }
              frame "T_8hr" {
                w373 = 28800.0  # 8 hours
                # "Time span selected: 4 hours"
                n125 = Unbundle By Name(w372) -> ("Time-End"=w371:timestamp)
                n126 = To Double Precision Float(number=w371) -> (double precision float=w377:dbl)
                n127 = Subtract(x=w377, y=w373) -> (x-y=w376:dbl)
                n128 = To Time Stamp(1:w376) -> (0:w375:timestamp)
                n129 = Bundle By Name(cluster=w372, "Time-Start"=w375, "TimeSpan(sec)"=w373) -> (w374:refnum<class "Gviewer.lvclass">)
              }
              frame "T_Today" {
                w389 = "%<%Y-%j>T" ("format string")
                # "Year + Day number"
                # "Time span selected: Since beginning of Today"
                n130 = Format Into String(format string=w389, error in=w387, w384) -> (resulting string=w388:string, error out=w386:errorcluster)  [unwired: 1 in]
                n131 = Scan From String(format string=w389, input string=w388, error in=w386) -> (error out=w385:errorcluster, output 1=w383:timestamp)  [unwired: 2 in, 2 out]
                n132 = To Double Precision Float(number=w384) -> (double precision float=w381:dbl)
                n133 = To Double Precision Float(number=w383) -> (double precision float=w380:dbl)
                n134 = Subtract(x=w381, y=w380) -> (x-y=w382:dbl)
                n135 = Bundle By Name(cluster=w390, "Live"=Typedef_Live."Live View", "Time-End"=w384, "Time-Start"=w383, "TimeSpan(sec)"=w382) -> (w391:refnum<class "Gviewer.lvclass">)
              }
              frame "T_month" {
                w402 = "%<%Y-%m>T" ("format string")
                # "Year + Month"
                # "Time span selected: Since beginning of this month"
                n136 = Format Into String(format string=w402, error in=w400, w397) -> (resulting string=w401:string, error out=w399:errorcluster)  [unwired: 1 in]
                n137 = Scan From String(format string=w402, input string=w401, error in=w399) -> (error out=w398:errorcluster, output 1=w396:timestamp)  [unwired: 2 in, 2 out]
                n138 = To Double Precision Float(number=w397) -> (double precision float=w394:dbl)
                n139 = To Double Precision Float(number=w396) -> (double precision float=w393:dbl)
                n140 = Subtract(x=w394, y=w393) -> (x-y=w395:dbl)
                n141 = Bundle By Name(cluster=w403, "Live"=Typedef_Live."Live View", "Time-End"=w397, "Time-Start"=w396, "TimeSpan(sec)"=w395) -> (w404:refnum<class "Gviewer.lvclass">)
              }
              frame "T_Year" {
                w415 = "%<%Y>T" ("format string")
                # "Time span selected: Since beginning of the Year"
                n142 = Format Into String(format string=w415, error in=w413, w410) -> (resulting string=w414:string, error out=w412:errorcluster)  [unwired: 1 in]
                n143 = Scan From String(format string=w415, input string=w414, error in=w412) -> (error out=w411:errorcluster, output 1=w409:timestamp)  [unwired: 2 in, 2 out]
                n144 = To Double Precision Float(number=w410) -> (double precision float=w407:dbl)
                n145 = To Double Precision Float(number=w409) -> (double precision float=w406:dbl)
                n146 = Subtract(x=w407, y=w406) -> (x-y=w408:dbl)
                n147 = Bundle By Name(cluster=w416, "Live"=Typedef_Live."Live View", "Time-End"=w410, "Time-Start"=w409, "TimeSpan(sec)"=w408) -> (w417:refnum<class "Gviewer.lvclass">)
              }
              frame "T_Week" {
                w428 = "%<%Y-%W>T" ("format string")
                # "Year + Week number"
                # "Time span selected: since beginning of this week"
                n148 = Format Into String(format string=w428, error in=w426, w423) -> (resulting string=w427:string, error out=w425:errorcluster)  [unwired: 1 in]
                n149 = Scan From String(format string=w428, input string=w427, error in=w425) -> (error out=w424:errorcluster, output 1=w422:timestamp)  [unwired: 2 in, 2 out]
                n150 = To Double Precision Float(number=w423) -> (double precision float=w420:dbl)
                n151 = To Double Precision Float(number=w422) -> (double precision float=w419:dbl)
                n152 = Subtract(x=w420, y=w419) -> (x-y=w421:dbl)
                n153 = Bundle By Name(cluster=w429, "Live"=Typedef_Live."Live View", "Time-End"=w423, "Time-Start"=w422, "TimeSpan(sec)"=w421) -> (w430:refnum<class "Gviewer.lvclass">)
              }
              frame "T_1day" {
                w433 = 86400.0  # 1 day
                # "Time span selected: 1 day"
                n154 = Unbundle By Name(w432) -> ("Time-End"=w431:timestamp)
                n155 = To Double Precision Float(number=w431) -> (double precision float=w437:dbl)
                n156 = Subtract(x=w437, y=w433) -> (x-y=w436:dbl)
                n157 = To Time Stamp(1:w436) -> (0:w435:timestamp)
                n158 = Bundle By Name(cluster=w432, "Time-Start"=w435, "TimeSpan(sec)"=w433) -> (w434:refnum<class "Gviewer.lvclass">)
              }
              frame "T_2days" {
                w441 = 172800.0  # 2 days
                # "Time span selected: 2 days"
                n159 = Unbundle By Name(w440) -> ("Time-End"=w439:timestamp)
                n160 = To Double Precision Float(number=w439) -> (double precision float=w445:dbl)
                n161 = Subtract(x=w445, y=w441) -> (x-y=w444:dbl)
                n162 = To Time Stamp(1:w444) -> (0:w443:timestamp)
                n163 = Bundle By Name(cluster=w440, "Time-Start"=w443, "TimeSpan(sec)"=w441) -> (w442:refnum<class "Gviewer.lvclass">)
              }
              frame "T_5days" {
                w449 = 432000.0  # 5 days
                # "Time span selected: 5 days"
                n164 = Unbundle By Name(w448) -> ("Time-End"=w447:timestamp)
                n165 = To Double Precision Float(number=w447) -> (double precision float=w453:dbl)
                n166 = Subtract(x=w453, y=w449) -> (x-y=w452:dbl)
                n167 = To Time Stamp(1:w452) -> (0:w451:timestamp)
                n168 = Bundle By Name(cluster=w448, "Time-Start"=w451, "TimeSpan(sec)"=w449) -> (w450:refnum<class "Gviewer.lvclass">)
              }
              frame "T_1wk" {
                w457 = 604800.0  # 7 days
                # "Time span selected: 1 week"
                n169 = Unbundle By Name(w456) -> ("Time-End"=w455:timestamp)
                n170 = To Double Precision Float(number=w455) -> (double precision float=w461:dbl)
                n171 = Subtract(x=w461, y=w457) -> (x-y=w460:dbl)
                n172 = To Time Stamp(1:w460) -> (0:w459:timestamp)
                n173 = Bundle By Name(cluster=w456, "Time-Start"=w459, "TimeSpan(sec)"=w457) -> (w458:refnum<class "Gviewer.lvclass">)
              }
              frame "T_2wks" {
                w465 = 1209600.0  # 14 days
                # "Time span selected: 2 weeks"
                n174 = Unbundle By Name(w464) -> ("Time-End"=w463:timestamp)
                n175 = To Double Precision Float(number=w463) -> (double precision float=w469:dbl)
                n176 = Subtract(x=w469, y=w465) -> (x-y=w468:dbl)
                n177 = To Time Stamp(1:w468) -> (0:w467:timestamp)
                n178 = Bundle By Name(cluster=w464, "Time-Start"=w467, "TimeSpan(sec)"=w465) -> (w466:refnum<class "Gviewer.lvclass">)
              }
              frame "T_1month" {
                w473 = 2678400.0  # 31 days
                # "Time span selected: one month"
                n179 = Unbundle By Name(w472) -> ("Time-End"=w471:timestamp)
                n180 = To Double Precision Float(number=w471) -> (double precision float=w477:dbl)
                n181 = Subtract(x=w477, y=w473) -> (x-y=w476:dbl)
                n182 = To Time Stamp(1:w476) -> (0:w475:timestamp)
                n183 = Bundle By Name(cluster=w472, "Time-Start"=w475, "TimeSpan(sec)"=w473) -> (w474:refnum<class "Gviewer.lvclass">)
              }
              frame "T_3months" {
                w481 = 7948800.0  # 92 days
                # "Time span selected: 1/4 Year"
                n184 = Unbundle By Name(w480) -> ("Time-End"=w479:timestamp)
                n185 = To Double Precision Float(number=w479) -> (double precision float=w485:dbl)
                n186 = Subtract(x=w485, y=w481) -> (x-y=w484:dbl)
                n187 = To Time Stamp(1:w484) -> (0:w483:timestamp)
                n188 = Bundle By Name(cluster=w480, "Time-Start"=w483, "TimeSpan(sec)"=w481) -> (w482:refnum<class "Gviewer.lvclass">)
              }
              frame "T_6months" {
                w489 = 15811200.0  # 183 days
                # "Time span selected: 1/2 Year"
                n189 = Unbundle By Name(w488) -> ("Time-End"=w487:timestamp)
                n190 = To Double Precision Float(number=w487) -> (double precision float=w493:dbl)
                n191 = Subtract(x=w493, y=w489) -> (x-y=w492:dbl)
                n192 = To Time Stamp(1:w492) -> (0:w491:timestamp)
                n193 = Bundle By Name(cluster=w488, "Time-Start"=w491, "TimeSpan(sec)"=w489) -> (w490:refnum<class "Gviewer.lvclass">)
              }
              frame "T_1year" {
                w497 = 31536000.0  # 365 days
                # "Time span selected: one Year"
                n194 = Unbundle By Name(w496) -> ("Time-End"=w495:timestamp)
                n195 = To Double Precision Float(number=w495) -> (double precision float=w501:dbl)
                n196 = Subtract(x=w501, y=w497) -> (x-y=w500:dbl)
                n197 = To Time Stamp(1:w500) -> (0:w499:timestamp)
                n198 = Bundle By Name(cluster=w496, "Time-Start"=w499, "TimeSpan(sec)"=w497) -> (w498:refnum<class "Gviewer.lvclass">)
              }
            }
            n199 = call "Request_Gserver_Update.vi"("error in (no error)"=w318, "Gviewer in"=w320) -> ("error out"=w317:errorcluster, "Gviewer out"=w319:refnum<class "Gviewer.lvclass">)  [unwired: 8 in]
            n200 = call "SetGraphTime.vi"("error in (no error)"=w317, "Gviewer in"=w319) -> ("error out"=w322:errorcluster, "Gviewer out"=w324:refnum<class "Gviewer.lvclass">)  [unwired: 8 in]
            n201 = call "GV_DrawLiveBox.vi"("error in (no error)"=w322, "Gviewer in"=w324) -> ("error out"=w321:errorcluster, "Gviewer out"=w323:refnum<class "Gviewer.lvclass">)  [unwired: 8 in]
          }
          frame "MenuCtx" {
            # "Options: Context menu"
            n202 = Unbundle By Name(w508) -> ("SettingsGeneral"=w513:T21)
            n203 = Unbundle By Name(w513) -> ("ContextMenu_active"=w514:bool, "MenuBar_active"=w511:bool)
            n204 = case shown="True" w514 {
              selector: w514 -> [w517 w519]
              tunnel: [w516 w521] -> w512
              tunnel: w511 -> [w515 w520]
              tunnel: [w515 w518] -> w510
              frame False {
                n205 = Not(x=w517) -> (.not. x?=w516:bool)
              }
              frame True {
                # "menu bar must be active\nif context menu is set to OFF"
                n206 = Or(x=w519, y=w520) -> (x .or. y?=w518:bool)
                n207 = Not(x=w519) -> (.not. x?=w521:bool)
              }
            }
            n208 = Bundle By Name(cluster=w513, "ContextMenu_active"=w512, "MenuBar_active"=w510) -> (w504:T21)
            n209 = Bundle By Name(cluster=w508, "SettingsGeneral"=w504) -> (w503:refnum<class "Gviewer.lvclass">)
            n210 = call "SendDataToServer.vi"("error in (no error)"=w505, "data"=w504, "Query_type"=Typedef_QueryType."SetClientOptions", "Gviewer in"=w503) -> ("error out"=w506:errorcluster, "Gviewer out"=w507:refnum<class "Gviewer.lvclass">)  [unwired: 6 in]
          }
          frame "ToolBare", "ToolGradient", "ToolNative" {
            # "Toolbar appearance layout change"
            n211 = case shown="\"ToolGradient\"" w525 {
              tunnel: [ToolBarAppearance."Native" ("ToolBarAppearance") ToolBarAppearance."Bare" ("ToolBarAppearance") ToolBarAppearance."Gradient" ("ToolBarAppearance")] -> w522
              frame Default {
              }
              frame "ToolBare" {
              }
              frame "ToolGradient" {
              }
            }
            n212 = Bundle By Name(cluster=w523, "ToolBarAppearance"=w522) -> (w524:refnum<class "Gviewer.lvclass">)
            n213 = call "GV_SetToolbar.vi"("error in (no error)"=w526, "Gviewer in"=w524) -> ("error out"=w527:errorcluster, "Gviewer out"=w528:refnum<class "Gviewer.lvclass">)  [unwired: 8 in]
          }
          frame "Pres_edit" {
            # "Open Preset Dialog"
            n214 = call "GV-StartPreset.vi"("error in (no error)"=w532, "Gviewer in"=w534) -> ("error out"=w533:errorcluster, "Gviewer out"=w535:refnum<class "Gviewer.lvclass">)  [unwired: 8 in]
          }
          frame "Pres_save" {
            # "Save current Preset setting"
            n215 = Unbundle By Name(w537) -> ("TagSelection"=w546:string[], "SelProperties"=w545:T10[])
            n216 = Unbundle By Name(w537) -> ("SettingsName"=w536:string)
            n217 = Unbundle By Name(w537) -> ("Settings_path"=w543:path)
            n218 = disable-structure shown="Enabled" {
              disable-tunnel: w543 -> [w564 w565]
              disable-tunnel: path "Presets" ("name or relative path") -> [w562 w567]
              disable-tunnel: [w561 w566] -> w539
              frame Enabled {
                # "One general presets path for all Graphs"
                n219 = Strip Path(path=w564) -> (stripped path=w563:path)  [unwired: 1 out]
                n220 = Build Path(base path=w563, name or relative path=w562) -> (appended path=w561:path)
              }
              frame Disabled {
                # "Specific settings per Graph instance"
                n221 = Build Path(base path=w565, name or relative path=w567) -> (appended path=w566:path)
              }
            }
            n222 = for {
              tunnel: w546 -> [w573] mode=indexing
              tunnel: w545 -> [w572] mode=indexing
              tunnel: [w568] -> w544 mode=indexing
              n223 = Unbundle By Name(w572) -> ("min"=w571:dbl, "max"=w570:dbl, "Color"=w569:u32)
              n224 = Bundle By Name(cluster=T8 {"TAG"="", "min"=0.0, "max"=0.0, "Color"=0} ("Selected-Tag"), "TAG"=w573, "min"=w571, "max"=w570, "Color"=w569) -> (w568:T8)
            }
            n225 = Unbundle By Name(w537) -> ("Live"=w548:T3)
            n226 = Equal?(x=Typedef_Live."Freeze" ("y"), y=w548) -> (x = y?=w549:bool)
            n227 = Concatenate Strings(w536, ".sgp" ("string")) -> (w541:string)
            n228 = Build Path(base path=w539, name or relative path=w541) -> (appended path=w538:path)
            n229 = Bundle By Name(cluster=T12 {"Save time?"=FALSE, "Presets"=[], "PresetFilePath"=path ""} ("PresetSave"), "Save time?"=w549, "Presets"=w544, "PresetFilePath"=w538) -> (w553:T12)
            n230 = Get Date/Time In Seconds() -> (seconds since 1Jan1904=w560:timestamp)
            n231 = To Variant(anything=w553) -> (Variant=w554:variant)
            n232 = Bundle By Name(cluster=T17 {"ServerActions"=enum."GraphUpdate", "data"=variant, "Source"="", "Time Stamp"=timestamp(0 s since 1904-01-01)} ("element"), "data"=w554, "ServerActions"=Typedef_ServerActions."EditTagsPresetSave", "Source"="Edit TAGs dialog", "Time Stamp"=w560) -> (w559:T17)
            n233 = Unbundle By Name(w537) -> ("GViewer-Queue"=w550:refnum<queue>)
            n234 = Enqueue Element(queue=w550, element=w559, error in (no error)=w551) -> (error out=w552:errorcluster)  [unwired: 1 in, 2 out]
          }
          frame "preset_0000".."preset_9999" {
            n235 = Unbundle By Name(w585) -> ("PresetsAvailable"=w587:string[])
            n236 = Match Pattern(string=w590, regular expression="preset_") -> (after substring=w588:string)  [unwired: 1 in, 3 out]
            n237 = Decimal String To Number(string=w588) -> (number=w586:i32)  [unwired: 2 in, 1 out]
            n238 = Index Array(array=w587, index=w586) -> (element=w584:string)
            n239 = call "Tag_settings_load.vi"("error in (no error)"=w581, "PresetName"=w584, "Gviewer in"=w585) -> ("error out"=w583:errorcluster, "Gviewer out"=w582:refnum<class "Gviewer.lvclass">)  [unwired: 7 in]
            n240 = call "SetMenuBar.vi"("error in (no error)"=w583, "Gviewer in"=w582) -> ("error out"=w576:errorcluster, "Gviewer out"=w579:refnum<class "Gviewer.lvclass">)  [unwired: 8 in]
            n241 = call "SetClassProperties.vi"("error in (no error)"=w576, "Gviewer in"=w579) -> ("error out"=w577:errorcluster, "Gviewer out"=w580:refnum<class "Gviewer.lvclass">)  [unwired: 8 in]
            n242 = call "Request_Gserver_Update.vi"("error in (no error)"=w577, "Gviewer in"=w580) -> ("error out"=w575:errorcluster, "Gviewer out"=w578:refnum<class "Gviewer.lvclass">)  [unwired: 8 in]
          }
          frame "Yscale_add" {
            # "Add an Y-axis to the graph"
            n243 = Unbundle By Name(w591) -> ("PlotSelected"=w597:i32)
            n244 = Greater Or Equal To 0?(x=w597) -> (x >= 0?=w596:bool)
            n245 = Select(t=ToolTypeEnum."41_AddYscalePlace" ("Enum"), s=w596, f=ToolTypeEnum."40_AddYscalePoint" ("Enum")) -> (s? t:f=w593:T18)
            n246 = Bundle By Name(cluster=w591, "ToolButtonSelected"=w593) -> (w592:refnum<class "Gviewer.lvclass">)
          }
          frame "Yscale_move" {
            # "Select an Y-scale for movement"
            n247 = Unbundle By Name(w599) -> ("PlotSelected"=w605:i32)
            n248 = Greater Or Equal To 0?(x=w605) -> (x >= 0?=w604:bool)
            n249 = Select(t=ToolTypeEnum."43_AddYscaleMoveDrag" ("Enum"), s=w604, f=ToolTypeEnum."42_AddYscaleMovePoint" ("Enum")) -> (s? t:f=w601:T18)
            n250 = Bundle By Name(cluster=w599, "ToolButtonSelected"=w601) -> (w600:refnum<class "Gviewer.lvclass">)
          }
          frame "Yscale_delete" {
            # "Delete an Y-scale"
            n251 = Unbundle By Name(w611) -> ("PlotSelected"=w607:i32)
            n252 = Greater Or Equal To 0?(x=w607) -> (x >= 0?=w610:bool)
            n253 = case shown="True" w610 {
              tunnel: [w616 w621] -> w612
              tunnel: w611 -> [w615 w623]
              tunnel: w609 -> [w613 w618]
              tunnel: [w613 w619] -> w608
              tunnel: w607 -> [_ w617]
              frame False {
                n254 = Bundle By Name(cluster=w615, "ToolButtonSelected"=ToolTypeEnum."44_AddYscaleDeletePoint" ("Enum")) -> (w616:refnum<class "Gviewer.lvclass">)
              }
              frame True {
                n255 = call "GV_YscaleDelete.vi"("error in (no error)"=w618, "Plot"=w617, "Gviewer in"=w623) -> ("error out"=w620:errorcluster, "Gviewer out"=w622:refnum<class "Gviewer.lvclass">)  [unwired: 7 in]
                n256 = call "GV_YscaleUpdateMenu.vi"("error in (no error)"=w620, "Gviewer in"=w622) -> ("error out"=w619:errorcluster, "Gviewer out"=w621:refnum<class "Gviewer.lvclass">)  [unwired: 8 in]
              }
            }
          }
          frame "Yscale_remove" {
            # "Remove all Y-scales"
            n257 = Initialize Array(T19 {"Plot"=0, "X(%)"=0.0} ("Ygraph"), 0 ("dimension size")) -> (w628:T19[])
            n258 = Bundle By Name(cluster=w631, "Yscales"=w628) -> (w627:refnum<class "Gviewer.lvclass">)
            n259 = call "GV_YscaleUpdateMenu.vi"("error in (no error)"=w624, "Gviewer in"=w627) -> ("error out"=w625:errorcluster, "Gviewer out"=w626:refnum<class "Gviewer.lvclass">)  [unwired: 8 in]
          }
          frame "YF0".."YF99" {
            # "Set Yscale resolution"
            n260 = String Subset(string=w645, offset (0)=2) -> (substring=w643:string)  [unwired: 1 in]
            n261 = Decimal String To Number(string=w643) -> (number=w636:i32)  [unwired: 2 in, 1 out]
            n262 = Bundle By Name(cluster=w642, "CurrentFormat"=w636) -> (w641:refnum<class "Gviewer.lvclass">)
            n263 = call "SetMenuBar.vi"("error in (no error)"=w640, "Gviewer in"=w641) -> ("error out"=w633:errorcluster, "Gviewer out"=w639:refnum<class "Gviewer.lvclass">)  [unwired: 8 in]
            n264 = Unbundle By Name(w639) -> ("Graph-ref"=w638:refnum<vi>, "YformatDefs"=w637:cluster{"Description":string, "Format":string}[])
            n265 = Index Array(array=w637, index=w636) -> (element=w635:cluster{"Description":string, "Format":string})
            n266 = Unbundle By Name(w635) -> ("Format"=w634:string)
            n267 = property class="XYGraph (strict)"(reference=w638, error in=w633, "YScale.FormatString"=w634) -> (error out=w632:errorcluster)  [unwired: 1 out]
          }
          frame "AutoMatch", "YscaleMatch" {
            # "Match Yscale units ON/OFF"
            n268 = Unbundle By Name(w646) -> ("YscaleMatch"=w649:bool)
            n269 = Not(x=w649) -> (.not. x?=w648:bool)
            n270 = Bundle By Name(cluster=w646, "YscaleMatch"=w648) -> (w647:refnum<class "Gviewer.lvclass">)
            n271 = call "SetMenuBar.vi"("error in (no error)"=w651, "Gviewer in"=w647) -> ("error out"=w650:errorcluster, "Gviewer out"=w652:refnum<class "Gviewer.lvclass">)  [unwired: 8 in]
          }
          frame "AutoContinuous" {
            # "Autoscale Continuous OFF"
            n272 = Unbundle By Name(w657) -> ("AutoscaleContinuous"=w659:bool)
            n273 = Not(x=w659) -> (.not. x?=w658:bool)
            n274 = Bundle By Name(cluster=w657, "AutoscaleContinuous"=w658) -> (w656:refnum<class "Gviewer.lvclass">)
            n275 = call "ToolBarButtonDraw.vi"("error in (no error)"=w653, "Gviewer in"=w656) -> ("error out"=w654:errorcluster, "Gviewer out"=w655:refnum<class "Gviewer.lvclass">)  [unwired: 8 in]
            n276 = call "SetMenuBar.vi"("error in (no error)"=w654, "Gviewer in"=w655) -> ("error out"=w660:errorcluster, "Gviewer out"=w661:refnum<class "Gviewer.lvclass">)  [unwired: 8 in]
          }
          frame "YscaleUseMinMax" {
            # "Autoscale Continuous OFF"
            n277 = Unbundle By Name(w666) -> ("YscaleUseMinMax"=w668:bool)
            n278 = Not(x=w668) -> (.not. x?=w667:bool)
            n279 = Bundle By Name(cluster=w666, "YscaleUseMinMax"=w667) -> (w665:refnum<class "Gviewer.lvclass">)
            n280 = call "ToolBarButtonDraw.vi"("error in (no error)"=w662, "Gviewer in"=w665) -> ("error out"=w663:errorcluster, "Gviewer out"=w664:refnum<class "Gviewer.lvclass">)  [unwired: 8 in]
            n281 = call "SetMenuBar.vi"("error in (no error)"=w663, "Gviewer in"=w664) -> ("error out"=w669:errorcluster, "Gviewer out"=w670:refnum<class "Gviewer.lvclass">)  [unwired: 8 in]
          }
          frame "CautoFitEq" {
            w672 = AutoScale."FitEqual" ("AutoScale")
            # "AutoScale action"
            n282 = Unbundle By Name(w676) -> ("GViewer-Queue"=w675:refnum<queue>)
            n283 = Bundle By Name(cluster=w676, "AutoScale"=w672, "AutoscaleContinuous"=TRUE) -> (w685:refnum<class "Gviewer.lvclass">)
            n284 = To Variant(anything=w672) -> (Variant=w671:variant)
            n285 = Get Date/Time In Seconds() -> (seconds since 1Jan1904=w673:timestamp)
            n286 = Bundle By Name(cluster=T17 {"ServerActions"=enum."GraphUpdate", "data"=variant, "Source"="", "Time Stamp"=timestamp(0 s since 1904-01-01)} ("element"), "ServerActions"=Typedef_ServerActions."AutoScale", "data"=w671, "Source"="MenuAction", "Time Stamp"=w673) -> (w679:T17)
            n287 = Enqueue Element(queue=w675, element=w679, error in (no error)=w678) -> (error out=w677:errorcluster)  [unwired: 1 in, 2 out]
            n288 = call "ToolBarButtonDraw.vi"("error in (no error)"=w677, "Gviewer in"=w685) -> ("error out"=w683:errorcluster, "Gviewer out"=w684:refnum<class "Gviewer.lvclass">)  [unwired: 8 in]
            n289 = call "SetMenuBar.vi"("error in (no error)"=w683, "Gviewer in"=w684) -> ("error out"=w686:errorcluster, "Gviewer out"=w687:refnum<class "Gviewer.lvclass">)  [unwired: 8 in]
          }
          frame "AutoFitEq" {
            w689 = AutoScale."FitEqual" ("AutoScale")
            # "AutoScale action"
            n290 = Unbundle By Name(w691) -> ("GViewer-Queue"=w698:refnum<queue>)
            n291 = Bundle By Name(cluster=w691, "AutoScale"=w689, "AutoscaleContinuous"=FALSE) -> (w701:refnum<class "Gviewer.lvclass">)
            n292 = To Variant(anything=w689) -> (Variant=w688:variant)
            n293 = Get Date/Time In Seconds() -> (seconds since 1Jan1904=w690:timestamp)
            n294 = Bundle By Name(cluster=T17 {"ServerActions"=enum."GraphUpdate", "data"=variant, "Source"="", "Time Stamp"=timestamp(0 s since 1904-01-01)} ("element"), "ServerActions"=Typedef_ServerActions."AutoScale", "data"=w688, "Source"="MenuAction", "Time Stamp"=w690) -> (w694:T17)
            n295 = Enqueue Element(queue=w698, element=w694, error in (no error)=w693) -> (error out=w692:errorcluster)  [unwired: 1 in, 2 out]
            n296 = call "ToolBarButtonDraw.vi"("error in (no error)"=w692, "Gviewer in"=w701) -> ("error out"=w699:errorcluster, "Gviewer out"=w700:refnum<class "Gviewer.lvclass">)  [unwired: 8 in]
            n297 = call "SetMenuBar.vi"("error in (no error)"=w699, "Gviewer in"=w700) -> ("error out"=w702:errorcluster, "Gviewer out"=w703:refnum<class "Gviewer.lvclass">)  [unwired: 8 in]
          }
          frame "CautoFitMax" {
            w706 = AutoScale."FitMax" ("AutoScale")
            # "AutoScale action"
            n298 = Unbundle By Name(w709) -> ("GViewer-Queue"=w716:refnum<queue>)
            n299 = Bundle By Name(cluster=w709, "AutoScale"=w706, "AutoscaleContinuous"=TRUE, "YscaleMatch"=FALSE ("AutoscaleContinuous")) -> (w719:refnum<class "Gviewer.lvclass">)
            n300 = To Variant(anything=w706) -> (Variant=w705:variant)
            n301 = Get Date/Time In Seconds() -> (seconds since 1Jan1904=w707:timestamp)
            n302 = Bundle By Name(cluster=T17 {"ServerActions"=enum."GraphUpdate", "data"=variant, "Source"="", "Time Stamp"=timestamp(0 s since 1904-01-01)} ("element"), "ServerActions"=Typedef_ServerActions."AutoScale", "data"=w705, "Source"="MenuAction", "Time Stamp"=w707) -> (w712:T17)
            n303 = Enqueue Element(queue=w716, element=w712, error in (no error)=w711) -> (error out=w710:errorcluster)  [unwired: 1 in, 2 out]
            n304 = call "ToolBarButtonDraw.vi"("error in (no error)"=w710, "Gviewer in"=w719) -> ("error out"=w717:errorcluster, "Gviewer out"=w718:refnum<class "Gviewer.lvclass">)  [unwired: 8 in]
            n305 = call "SetMenuBar.vi"("error in (no error)"=w717, "Gviewer in"=w718) -> ("error out"=w720:errorcluster, "Gviewer out"=w721:refnum<class "Gviewer.lvclass">)  [unwired: 8 in]
          }
          frame "AutoFitMax" {
            w726 = FALSE ("AutoscaleContinuous")
            w724 = AutoScale."FitMax" ("AutoScale")
            # "AutoScale action"
            n306 = Unbundle By Name(w727) -> ("GViewer-Queue"=w734:refnum<queue>)
            n307 = To Variant(anything=w724) -> (Variant=w723:variant)
            n308 = Bundle By Name(cluster=w727, "AutoScale"=w724, "AutoscaleContinuous"=w726, "YscaleMatch"=w726) -> (w737:refnum<class "Gviewer.lvclass">)
            n309 = Get Date/Time In Seconds() -> (seconds since 1Jan1904=w725:timestamp)
            n310 = Bundle By Name(cluster=T17 {"ServerActions"=enum."GraphUpdate", "data"=variant, "Source"="", "Time Stamp"=timestamp(0 s since 1904-01-01)} ("element"), "ServerActions"=Typedef_ServerActions."AutoScale", "data"=w723, "Source"="MenuAction", "Time Stamp"=w725) -> (w730:T17)
            n311 = Enqueue Element(queue=w734, element=w730, error in (no error)=w729) -> (error out=w728:errorcluster)  [unwired: 1 in, 2 out]
            n312 = call "ToolBarButtonDraw.vi"("error in (no error)"=w728, "Gviewer in"=w737) -> ("error out"=w735:errorcluster, "Gviewer out"=w736:refnum<class "Gviewer.lvclass">)  [unwired: 8 in]
            n313 = call "SetMenuBar.vi"("error in (no error)"=w735, "Gviewer in"=w736) -> ("error out"=w738:errorcluster, "Gviewer out"=w739:refnum<class "Gviewer.lvclass">)  [unwired: 8 in]
          }
          frame "CautoStackEq" {
            w741 = AutoScale."StackEqual" ("AutoScale")
            # "AutoScale action"
            n314 = Unbundle By Name(w743) -> ("GViewer-Queue"=w750:refnum<queue>)
            n315 = To Variant(anything=w741) -> (Variant=w740:variant)
            n316 = Bundle By Name(cluster=w743, "AutoScale"=w741, "AutoscaleContinuous"=TRUE) -> (w753:refnum<class "Gviewer.lvclass">)
            n317 = Get Date/Time In Seconds() -> (seconds since 1Jan1904=w742:timestamp)
            n318 = Bundle By Name(cluster=T17 {"ServerActions"=enum."GraphUpdate", "data"=variant, "Source"="", "Time Stamp"=timestamp(0 s since 1904-01-01)} ("element"), "ServerActions"=Typedef_ServerActions."AutoScale", "data"=w740, "Source"="MenuAction", "Time Stamp"=w742) -> (w746:T17)
            n319 = Enqueue Element(queue=w750, element=w746, error in (no error)=w745) -> (error out=w744:errorcluster)  [unwired: 1 in, 2 out]
            n320 = call "ToolBarButtonDraw.vi"("error in (no error)"=w744, "Gviewer in"=w753) -> ("error out"=w751:errorcluster, "Gviewer out"=w752:refnum<class "Gviewer.lvclass">)  [unwired: 8 in]
            n321 = call "SetMenuBar.vi"("error in (no error)"=w751, "Gviewer in"=w752) -> ("error out"=w754:errorcluster, "Gviewer out"=w755:refnum<class "Gviewer.lvclass">)  [unwired: 8 in]
          }
          frame "AutoStackEq" {
            w758 = AutoScale."StackEqual" ("AutoScale")
            # "AutoScale action"
            n322 = Unbundle By Name(w760) -> ("GViewer-Queue"=w767:refnum<queue>)
            n323 = Bundle By Name(cluster=w760, "AutoScale"=w758, "AutoscaleContinuous"=FALSE) -> (w770:refnum<class "Gviewer.lvclass">)
            n324 = To Variant(anything=w758) -> (Variant=w757:variant)
            n325 = Get Date/Time In Seconds() -> (seconds since 1Jan1904=w759:timestamp)
            n326 = Bundle By Name(cluster=T17 {"ServerActions"=enum."GraphUpdate", "data"=variant, "Source"="", "Time Stamp"=timestamp(0 s since 1904-01-01)} ("element"), "ServerActions"=Typedef_ServerActions."AutoScale", "data"=w757, "Source"="MenuAction", "Time Stamp"=w759) -> (w763:T17)
            n327 = Enqueue Element(queue=w767, element=w763, error in (no error)=w762) -> (error out=w761:errorcluster)  [unwired: 1 in, 2 out]
            n328 = call "ToolBarButtonDraw.vi"("error in (no error)"=w761, "Gviewer in"=w770) -> ("error out"=w768:errorcluster, "Gviewer out"=w769:refnum<class "Gviewer.lvclass">)  [unwired: 8 in]
            n329 = call "SetMenuBar.vi"("error in (no error)"=w768, "Gviewer in"=w769) -> ("error out"=w771:errorcluster, "Gviewer out"=w772:refnum<class "Gviewer.lvclass">)  [unwired: 8 in]
          }
          frame "AutoStackType" {
            w775 = AutoScale."StackPerType" ("AutoScale")
            # "AutoScale action"
            n330 = Unbundle By Name(w777) -> ("GViewer-Queue"=w784:refnum<queue>)
            n331 = Bundle By Name(cluster=w777, "AutoScale"=w775, "AutoscaleContinuous"=FALSE) -> (w787:refnum<class "Gviewer.lvclass">)
            n332 = To Variant(anything=w775) -> (Variant=w774:variant)
            n333 = Get Date/Time In Seconds() -> (seconds since 1Jan1904=w776:timestamp)
            n334 = Bundle By Name(cluster=T17 {"ServerActions"=enum."GraphUpdate", "data"=variant, "Source"="", "Time Stamp"=timestamp(0 s since 1904-01-01)} ("element"), "ServerActions"=Typedef_ServerActions."AutoScale", "data"=w774, "Source"="MenuAction", "Time Stamp"=w776) -> (w780:T17)
            n335 = Enqueue Element(queue=w784, element=w780, error in (no error)=w779) -> (error out=w778:errorcluster)  [unwired: 1 in, 2 out]
            n336 = call "ToolBarButtonDraw.vi"("error in (no error)"=w778, "Gviewer in"=w787) -> ("error out"=w785:errorcluster, "Gviewer out"=w786:refnum<class "Gviewer.lvclass">)  [unwired: 8 in]
            n337 = call "SetMenuBar.vi"("error in (no error)"=w785, "Gviewer in"=w786) -> ("error out"=w788:errorcluster, "Gviewer out"=w789:refnum<class "Gviewer.lvclass">)  [unwired: 8 in]
          }
          frame "CautoStackMax" {
            w792 = AutoScale."StackMax" ("AutoScale")
            # "AutoScale action"
            n338 = Unbundle By Name(w795) -> ("GViewer-Queue"=w802:refnum<queue>)
            n339 = Bundle By Name(cluster=w795, "AutoScale"=w792, "AutoscaleContinuous"=TRUE, "YscaleMatch"=FALSE ("AutoscaleContinuous")) -> (w805:refnum<class "Gviewer.lvclass">)
            n340 = To Variant(anything=w792) -> (Variant=w791:variant)
            n341 = Get Date/Time In Seconds() -> (seconds since 1Jan1904=w793:timestamp)
            n342 = Bundle By Name(cluster=T17 {"ServerActions"=enum."GraphUpdate", "data"=variant, "Source"="", "Time Stamp"=timestamp(0 s since 1904-01-01)} ("element"), "ServerActions"=Typedef_ServerActions."AutoScale", "data"=w791, "Source"="MenuAction", "Time Stamp"=w793) -> (w798:T17)
            n343 = Enqueue Element(queue=w802, element=w798, error in (no error)=w797) -> (error out=w796:errorcluster)  [unwired: 1 in, 2 out]
            n344 = call "ToolBarButtonDraw.vi"("error in (no error)"=w796, "Gviewer in"=w805) -> ("error out"=w803:errorcluster, "Gviewer out"=w804:refnum<class "Gviewer.lvclass">)  [unwired: 8 in]
            n345 = call "SetMenuBar.vi"("error in (no error)"=w803, "Gviewer in"=w804) -> ("error out"=w806:errorcluster, "Gviewer out"=w807:refnum<class "Gviewer.lvclass">)  [unwired: 8 in]
          }
          frame "CautoStackType" {
            w810 = AutoScale."StackPerType" ("AutoScale")
            # "AutoScale action"
            n346 = Unbundle By Name(w813) -> ("GViewer-Queue"=w820:refnum<queue>)
            n347 = Bundle By Name(cluster=w813, "AutoScale"=w810, "AutoscaleContinuous"=TRUE, "YscaleMatch"=FALSE ("AutoscaleContinuous")) -> (w823:refnum<class "Gviewer.lvclass">)
            n348 = To Variant(anything=w810) -> (Variant=w809:variant)
            n349 = Get Date/Time In Seconds() -> (seconds since 1Jan1904=w811:timestamp)
            n350 = Bundle By Name(cluster=T17 {"ServerActions"=enum."GraphUpdate", "data"=variant, "Source"="", "Time Stamp"=timestamp(0 s since 1904-01-01)} ("element"), "ServerActions"=Typedef_ServerActions."AutoScale", "data"=w809, "Source"="MenuAction", "Time Stamp"=w811) -> (w816:T17)
            n351 = Enqueue Element(queue=w820, element=w816, error in (no error)=w815) -> (error out=w814:errorcluster)  [unwired: 1 in, 2 out]
            n352 = call "ToolBarButtonDraw.vi"("error in (no error)"=w814, "Gviewer in"=w823) -> ("error out"=w821:errorcluster, "Gviewer out"=w822:refnum<class "Gviewer.lvclass">)  [unwired: 8 in]
            n353 = call "SetMenuBar.vi"("error in (no error)"=w821, "Gviewer in"=w822) -> ("error out"=w824:errorcluster, "Gviewer out"=w825:refnum<class "Gviewer.lvclass">)  [unwired: 8 in]
          }
          frame "AutoStackMax" {
            w830 = FALSE ("AutoscaleContinuous")
            w828 = AutoScale."StackMax" ("AutoScale")
            # "AutoScale action"
            n354 = Unbundle By Name(w832) -> ("GViewer-Queue"=w838:refnum<queue>)
            n355 = To Variant(anything=w828) -> (Variant=w827:variant)
            n356 = Bundle By Name(cluster=w832, "AutoScale"=w828, "AutoscaleContinuous"=w830, "YscaleMatch"=w830) -> (w841:refnum<class "Gviewer.lvclass">)
            n357 = Get Date/Time In Seconds() -> (seconds since 1Jan1904=w829:timestamp)
            n358 = Bundle By Name(cluster=T17 {"ServerActions"=enum."GraphUpdate", "data"=variant, "Source"="", "Time Stamp"=timestamp(0 s since 1904-01-01)} ("element"), "ServerActions"=Typedef_ServerActions."AutoScale", "data"=w827, "Source"="MenuAction", "Time Stamp"=w829) -> (w834:T17)
            n359 = Enqueue Element(queue=w838, element=w834, error in (no error)=w833) -> (error out=w831:errorcluster)  [unwired: 1 in, 2 out]
            n360 = call "ToolBarButtonDraw.vi"("error in (no error)"=w831, "Gviewer in"=w841) -> ("error out"=w839:errorcluster, "Gviewer out"=w840:refnum<class "Gviewer.lvclass">)  [unwired: 8 in]
            n361 = call "SetMenuBar.vi"("error in (no error)"=w839, "Gviewer in"=w840) -> ("error out"=w842:errorcluster, "Gviewer out"=w843:refnum<class "Gviewer.lvclass">)  [unwired: 8 in]
          }
          frame "DBedit" {
            # "Start the database Editor"
            n362 = call "GV_StartDBeditor.vi"("error in (no error)"=w845, "Gviewer in"=w847) -> ("error out"=w844:errorcluster, "Gviewer out"=w846:refnum<class "Gviewer.lvclass">)  [unwired: 8 in]
          }
          frame "MinMaxFocus", "MinMaxOff", "MinMaxOn" {
            # "MinMax setting"
            n363 = case shown="\"MinMaxFocus\"" w854 {
              tunnel: [MinMax."Off" ("MinMax") MinMax."On" ("MinMax") MinMax."Off" ("MinMax") MinMax."Focus" ("MinMax")] -> w850
              frame Default {
              }
              frame "MinMaxOn" {
              }
              frame "MinMaxOff" {
              }
              frame "MinMaxFocus" {
              }
            }
            n364 = Bundle By Name(cluster=w848, "MinMax"=w850) -> (w849:refnum<class "Gviewer.lvclass">)
            n365 = call "SetMenuBar.vi"("error in (no error)"=w852, "Gviewer in"=w849) -> ("error out"=w851:errorcluster, "Gviewer out"=w853:refnum<class "Gviewer.lvclass">)  [unwired: 8 in]
          }
          frame Default {
            n366 = Concatenate Strings("Menu item not implemented:\n", w862) -> (w861:string)
            n367 = One Button Dialog(message=w861) -> ()  [unwired: 1 in, 1 out]
          }
        }
        n368 = disable-structure shown="Disabled" {
          frame Disabled {
            (unwired) ToolTypeEnum."21_VerticalMove" ("Enum")
          }
          frame Enabled {
          }
        }
      }
      event Pane Size {
        # "Rearange all objects to Pane size"
        n369 = event-data() -> ()  [unwired: 1 in, 3 out]
        n370 = call "GV_SetToolbar.vi"("error in (no error)"=w877, "Gviewer in"=w878) -> ("error out"=w875:errorcluster, "Gviewer out"=w876:refnum<class "Gviewer.lvclass">)  [unwired: 8 in]
        n371 = call "GV_SetGraph.vi"("error in (no error)"=w875, "Gviewer in"=w876) -> ("error out"=w873:errorcluster, "Gviewer out"=w874:refnum<class "Gviewer.lvclass">)  [unwired: 8 in]
        n372 = call "GV_DrawLiveBox.vi"("error in (no error)"=w873, "Gviewer in"=w874) -> ("error out"=w868:errorcluster, "Gviewer out"=w869:refnum<class "Gviewer.lvclass">)  [unwired: 8 in]
        n373 = call "GV_timedToolButtonsUpdate.vi"("error in (no error)"=w868, "Gviewer in"=w869) -> ("error out"=w865:errorcluster, "Gviewer out"=w867:refnum<class "Gviewer.lvclass">)  [unwired: 8 in]
        n374 = call "GV_timedGraphRequestUpdate.vi"("error in (no error)"=w865, "Gviewer in"=w867) -> ("error out"=w864:errorcluster, "Gviewer out"=w866:refnum<class "Gviewer.lvclass">)  [unwired: 8 in]
        n375 = Unbundle By Name(w866) -> ("Visible"=w872:bool)
        n376 = case shown="True" w872 {
          tunnel: w866 -> [w880 w881]
          tunnel: [w880 w882] -> w871
          tunnel: w864 -> [w879 w883]
          tunnel: [w879 w884] -> w870
          frame False {
          }
          frame True {
            n377 = Unbundle By Name(w881) -> ("Graph-ref"=w886:refnum<vi>)
            n378 = property class="XYGraph (strict)"(reference=w886, error in=w883) -> (error out=w884:errorcluster, "LegPos"=w885:T22)  [unwired: 1 out]
            n379 = Bundle By Name(cluster=w881, "Position"=w885) -> (w882:refnum<class "Gviewer.lvclass">)
          }
        }
      }
      event "Graph": Mouse Move {
        # "Draw cursor info when mouse is moved"
        n380 = event-data() -> ("Coords"=w888:T23)  [unwired: 1 in]
        n381 = call "CursorDraw.vi"("error in (no error)"=w893, "Coords"=w888, "Gviewer in"=w889) -> ("error out"=w891:errorcluster, "Gviewer out"=w892:refnum<class "Gviewer.lvclass">)  [unwired: 7 in]
        n382 = call "GV_timedToolButtonsUpdate.vi"("error in (no error)"=w891, "Gviewer in"=w892) -> ("error out"=w890:errorcluster, "Gviewer out"=w887:refnum<class "Gviewer.lvclass">)  [unwired: 8 in]
      }
      event "Graph": Mouse Down {
        # "Click on a mouse button when on the graph"
        n383 = event-data() -> ("Button"=w895:u16, "Coords"=w896:T23)  [unwired: 1 in]
        n384 = call "GV-MouseDown.vi"("error in (no error)"=w897, "Coords"=w896, "Button"=w895, "Gviewer in"=w899) -> ("error out"=w898:errorcluster, "Gviewer out"=w894:refnum<class "Gviewer.lvclass">)  [unwired: 6 in]
      }
      event "Graph": Mouse Up {
        # "Release mouse while hovering over graph"
        n385 = event-data() -> ("Coords"=w901:T23)  [unwired: 1 in]
        n386 = call "GV-MouseUP.vi"("MouseLeave?"=FALSE, "error in (no error)"=w902, "Coords"=w901, "Gviewer in"=w904) -> ("error out"=w903:errorcluster, "Gviewer out"=w905:refnum<class "Gviewer.lvclass">)  [unwired: 6 in]
      }
      event "Graph": Mouse Wheel {
        # "Mouse scroll zoom functions"
        n387 = event-data() -> ("Coords"=w906:T23, "Delta"=w907:i32)  [unwired: 1 in]
        n388 = Unbundle By Name(w911) -> ("ToolButtonSelected"=w912:i32)
        n389 = case shown="22" w912 {
          tunnel: w911 -> [w914 w926 w941]
          tunnel: w910 -> [w913 w925 w938]
          tunnel: [w914 w917 w929] -> w909
          tunnel: [w913 w916 w928] -> w908
          tunnel: w907 -> [_ w924 w939]
          tunnel: w906 -> [_ w923 w940]
          frame Default {
            # "Not identified"
          }
          frame 20 {
            w915 = FALSE  # F = When scrolling is done
            # "Vertical Scroll zoom"
            n390 = call "Scroll-Vzoom.vi"("error in (no error)"=w925, "Scroll value"=w924, "Coords"=w923, "Gviewer in"=w926) -> ("error out"=w922:errorcluster, "Gviewer out"=w921:refnum<class "Gviewer.lvclass">)  [unwired: 6 in]
            n391 = Unbundle By Name(w921) -> ("LastUpdate"=w920:T4)
            n392 = call "GV-SetGraphData.vi"("error in (no error)"=w922, "GviewerUpdate"=w920, "Gviewer in"=w921) -> ("error out"=w918:errorcluster, "Gviewer out"=w919:refnum<class "Gviewer.lvclass">)  [unwired: 7 in]
            n393 = call "GV_StoreNewZoomValue.vi"("Immediate"=w915, "error in (no error)"=w918, "Gviewer in"=w919) -> ("error out"=w916:errorcluster, "Gviewer out"=w917:refnum<class "Gviewer.lvclass">)  [unwired: 7 in]
          }
          frame 22 {
            w927 = FALSE  # F = when scrolling is done
            # "Time zoom"
            n394 = call "Scroll-Hzoom.vi"("error in (no error)"=w938, "Scroll value"=w939, "Coords"=w940, "Gviewer in"=w941) -> ("error out"=w932:errorcluster, "Gviewer out"=w935:refnum<class "Gviewer.lvclass">)  [unwired: 6 in]
            n395 = call "Request_Gserver_Update.vi"("error in (no error)"=w932, "Gviewer in"=w935) -> ("error out"=w936:errorcluster, "Gviewer out"=w937:refnum<class "Gviewer.lvclass">)  [unwired: 8 in]
            n396 = call "SetGraphTime.vi"("error in (no error)"=w936, "Gviewer in"=w937) -> ("error out"=w934:errorcluster, "Gviewer out"=w933:refnum<class "Gviewer.lvclass">)  [unwired: 8 in]
            n397 = call "GV_ToolbarShowTimeSpan.vi"("error in (no error)"=w934, "Gviewer in"=w933) -> ("error out"=w931:errorcluster, "Gviewer out"=w930:refnum<class "Gviewer.lvclass">)  [unwired: 7 in, 1 out]
            n398 = call "GV_StoreNewZoomValue.vi"("Immediate"=w927, "error in (no error)"=w931, "Gviewer in"=w930) -> ("error out"=w928:errorcluster, "Gviewer out"=w929:refnum<class "Gviewer.lvclass">)  [unwired: 7 in]
          }
        }
      }
      event "Graph": Mouse Leave {
        # "Sanity actions when leaving the graph area with mouse"
        n399 = event-data() -> ()  [unwired: 1 in, 1 out]
        n400 = call "GV-MouseUP.vi"("MouseLeave?"=TRUE, "error in (no error)"=w943, "Gviewer in"=w945) -> ("error out"=w944:errorcluster, "Gviewer out"=w946:refnum<class "Gviewer.lvclass">)  [unwired: 7 in]
      }
      event Key Down {
        # "Press a key"
        n401 = event-data() -> ("ScanCode"=w954:i16, "VKey"=w962:T2, "PlatMods.Shift"=w961:bool, "PlatMods.Ctrl"=w960:bool)  [unwired: 1 in]
        n402 = Unbundle By Name(w957) -> ("KeyStrokes_Lookup"=w964:i16[])
        n403 = Get Date/Time In Seconds() -> (seconds since 1Jan1904=w959:timestamp)
        n404 = Search 1D Array(1D array=w964, element=w954) -> (index of element=w958:i32)  [unwired: 1 in]
        n405 = Bundle By Name(cluster=T1 {"Char"=0, "VKey"=enum."ASCII", "Shift"=FALSE, "Ctrl"=FALSE, "Time"=timestamp(0 s since 1904-01-01)} ("Key"), "Char"=w954, "VKey"=w962, "Shift"=w961, "Ctrl"=w960, "Time"=w959) -> (w955:T1)
        n406 = case shown="-1" w958 {
          selector: w958 -> [w971 _]
          tunnel: w957 -> [w965 w985]
          tunnel: w956 -> [w974 w976]
          tunnel: [w974 w977] -> w953
          tunnel: [w966 w978] -> w948
          tunnel: w955 -> [w970 w975]
          tunnel: w954 -> [w969 w982]
          frame Default {
            # "Replace if the switch action already exists"
            n407 = Unbundle By Name(w965) -> ("KeyStrokes_Lookup"=w973:i16[], "KeyStrokes"=w972:T1[])
            n408 = Replace Array Subset(array=w973, new element=w969, index=w971) -> (w968:i16[])
            n409 = Replace Array Subset(array=w972, new element=w970, index=w971) -> (w967:T1[])
            n410 = Bundle By Name(cluster=w965, "KeyStrokes_Lookup"=w968, "KeyStrokes"=w967) -> (w966:refnum<class "Gviewer.lvclass">)
          }
          frame -1 {
            # "Actions on switch pressing\nare in here"
            # "New switch pressure"
            n411 = Unbundle By Name(w985) -> ("KeyStrokes_Lookup"=w984:i16[], "KeyStrokes"=w981:T1[])
            n412 = Build Array (concatenate)(w981, w975) -> (w980:T1[])
            n413 = Build Array (concatenate)(w984, w982) -> (w983:i16[])
            n414 = Bundle By Name(cluster=w985, "KeyStrokes_Lookup"=w983, "KeyStrokes"=w980) -> (w979:refnum<class "Gviewer.lvclass">)
            n415 = call "KeySwitched.vi"("error in (no error)"=w976, "Key"=w975, "Gviewer in"=w979) -> ("error out"=w977:errorcluster, "Gviewer out"=w978:refnum<class "Gviewer.lvclass">)  [unwired: 6 in, 1 out]
            "Key DN" <- w975
          }
        }
        n416 = Unbundle By Name(w948) -> ("GraphCursorLoc"=w947:T23)
        n417 = call "ToolBarButtonDraw.vi"("error in (no error)"=w953, "Gviewer in"=w948) -> ("error out"=w951:errorcluster, "Gviewer out"=w949:refnum<class "Gviewer.lvclass">)  [unwired: 8 in]
        n418 = call "CursorDraw.vi"("error in (no error)"=w951, "Coords"=w947, "Gviewer in"=w949) -> ("error out"=w950:errorcluster, "Gviewer out"=w952:refnum<class "Gviewer.lvclass">)  [unwired: 7 in]
      }
      event Key Up {
        # "Release a key"
        n419 = event-data() -> ("ScanCode"=w993:i16)  [unwired: 1 in]
        n420 = Unbundle By Name(w996) -> ("KeyStrokes_Lookup"=w994:i16[])
        n421 = Search 1D Array(1D array=w994, element=w993) -> (index of element=w997:i32)  [unwired: 1 in]
        n422 = case shown="Default" w997 {
          selector: w997 -> [w1006 _]
          tunnel: w996 -> [w1007 w1013]
          tunnel: w995 -> [w999 w1012]
          tunnel: [w1004 w1013] -> w986
          tunnel: [w1000 w1012] -> w988
          frame Default {
            w1002 = 1 ("index")
            n423 = Unbundle By Name(w1007) -> ("KeyStrokes_Lookup"=w1011:i16[], "KeyStrokes"=w1010:T1[])
            n424 = Delete From Array(array=w1011, length=w1002, index=w1006) -> (array with subset deleted=w1009:i16[])  [unwired: 1 out]
            n425 = Delete From Array(array=w1010, length=w1002, index=w1006) -> (deleted portion=w1003:T1[], array with subset deleted=w1008:T1[])
            n426 = Bundle By Name(cluster=w1007, "KeyStrokes_Lookup"=w1009, "KeyStrokes"=w1008) -> (w1005:refnum<class "Gviewer.lvclass">)
            n427 = Index Array(array=w1003, index=0) -> (element=w1001:T1)
            "Key UP" <- w1001
            n428 = call "KeyUnSwitched.vi"("error in (no error)"=w999, "Key"=w1001, "Gviewer in"=w1005) -> ("error out"=w1000:errorcluster, "Gviewer out"=w1004:refnum<class "Gviewer.lvclass">)  [unwired: 7 in]
          }
          frame -1 {
          }
        }
        n429 = Unbundle By Name(w986) -> ("GraphCursorLoc"=w991:T23)
        n430 = call "ToolBarButtonDraw.vi"("error in (no error)"=w988, "Gviewer in"=w986) -> ("error out"=w989:errorcluster, "Gviewer out"=w992:refnum<class "Gviewer.lvclass">)  [unwired: 8 in]
        n431 = call "CursorDraw.vi"("error in (no error)"=w989, "Coords"=w991, "Gviewer in"=w992) -> ("error out"=w987:errorcluster, "Gviewer out"=w990:refnum<class "Gviewer.lvclass">)  [unwired: 7 in]
      }
      event Mouse Up {
        # "Detect mouse up event (after dragging action)"
        n432 = event-data() -> ("Coords"=w1015:T23)  [unwired: 1 in]
        n433 = call "GV-MouseUP.vi"("MouseLeave?"=FALSE, "error in (no error)"=w1016, "Coords"=w1015, "Gviewer in"=w1018) -> ("error out"=w1017:errorcluster, "Gviewer out"=w1019:refnum<class "Gviewer.lvclass">)  [unwired: 6 in]
      }
      event "ToolBar": Mouse Move {
        # "Update toolbar icons when hovering over it"
        n434 = event-data() -> ("Coords"=w1024:T23)  [unwired: 1 in]
        n435 = call "ToolBarButtonDraw.vi"("error in (no error)"=w1025, "Coords"=w1024, "Gviewer in"=w1026) -> ("error out"=w1021:errorcluster, "Gviewer out"=w1023:refnum<class "Gviewer.lvclass">)  [unwired: 7 in]
        n436 = call "GV_ToolbarShowTimeSpan.vi"("error in (no error)"=w1021, "Gviewer in"=w1023) -> ("error out"=w1020:errorcluster, "Gviewer out"=w1022:refnum<class "Gviewer.lvclass">)  [unwired: 7 in, 1 out]
      }
      event "ToolBar": Mouse Down {
        # "Press a button on the toolbar"
        n437 = event-data() -> ("Coords"=w1027:T23)  [unwired: 1 in]
        n438 = Unbundle By Name(w1035) -> ("ToolButtonFocus"=w1032:i32)
        n439 = Bundle By Name(cluster=w1035, "ToolButtonSelected"=w1032) -> (w1034:refnum<class "Gviewer.lvclass">)
        n440 = call "ToolBarButtonDraw.vi"("error in (no error)"=w1033, "Coords"=w1027, "Gviewer in"=w1034) -> ("error out"=w1031:errorcluster, "Gviewer out"=w1029:refnum<class "Gviewer.lvclass">)  [unwired: 7 in]
        n441 = case shown="4" w1032 {
          selector: w1032 -> [_ _ _ w1058 w1062 _ _]
          tunnel: w1031 -> [w1037 w1042 w1055 w1057 w1061 w1078 w1094]
          tunnel: [w1037 w1041 w1053 w1057 w1061 w1077 w1093] -> w1030
          tunnel: w1029 -> [w1036 w1040 w1056 w1060 w1064 w1071 w1089]
          tunnel: [w1036 w1039 w1054 w1059 w1063 w1082 w1100] -> w1028
          tunnel: w1027 -> [_ _ w1052 _ _ _ _]
          frame Default {
          }
          frame 0 {
            w1038 = -1  # Remove Selection
            # "Escape"
            n442 = Unbundle By Name(w1040) -> ("TagSelection"=w1043:string[], "Graph-ref"=w1044:refnum<vi>)
            n443 = for {
              tunnel: w1044 -> [w1051]
              shift-right: [w1047] -> w1041
              shift-left: w1042 -> [w1049]
              tunnel: w1043 -> [_] mode=indexing
              i -> [w1046]
              # "Remove any trace selection"
              n444 = property class="XYGraph (strict)"(reference=w1051, error in=w1049, "Active Plot"=w1046) -> (reference out=w1050:refnum<vi>, error out=w1048:errorcluster)
              n445 = property class="XYGraph (strict)"(reference=w1050, error in=w1048, "Plot.Line Width"=u8 1) -> (error out=w1047:errorcluster)  [unwired: 1 out]
            }
            n446 = Bundle By Name(cluster=w1040, "PlotSelected"=w1038, "PrevToolButton"=w1038) -> (w1039:refnum<class "Gviewer.lvclass">)
          }
          frame 1 {
            # "Undo"
            n447 = call "GV_undo.vi"("error in (no error)"=w1055, "Coords"=w1052, "Gviewer in"=w1056) -> ("error out"=w1053:errorcluster, "Gviewer out"=w1054:refnum<class "Gviewer.lvclass">)  [unwired: 7 in]
          }
          frame 2 {
            # "Help"
            n448 = Bundle By Name(cluster=w1060, "PrevToolButton"=w1058) -> (w1059:refnum<class "Gviewer.lvclass">)
          }
          frame 3 {
            # "Cursor"
            n449 = Bundle By Name(cluster=w1064, "PrevToolButton"=w1062) -> (w1063:refnum<class "Gviewer.lvclass">)
          }
          frame 4 {
            # "Autoscale Fit"
            n450 = Unbundle By Name(w1071) -> ("YscaleMatch"=w1066:bool, "PrevToolButton"=w1079:i32, "GViewer-Queue"=w1076:refnum<queue>)
            n451 = Get Date/Time In Seconds() -> (seconds since 1Jan1904=w1072:timestamp)
            n452 = Select(t=AutoScale."FitEqual" ("AutoScale"), s=w1066, f=AutoScale."FitMax" ("AutoScale")) -> (s? t:f=w1065:T13)
            n453 = To Variant(anything=w1065) -> (Variant=w1069:variant)
            n454 = To Double Precision Float(number=w1072) -> (double precision float=w1080:dbl)
            n455 = Bundle By Name(cluster=T17 {"ServerActions"=enum."GraphUpdate", "data"=variant, "Source"="", "Time Stamp"=timestamp(0 s since 1904-01-01)} ("element"), "ServerActions"=Typedef_ServerActions."AutoScale", "data"=w1069, "Source"="Toolbar", "Time Stamp"=w1072) -> (w1074:T17)
            n456 = Bundle By Name(cluster=w1071, "AutoScale"=w1065, "AutoscaleContinuous"=FALSE, "ContOnTimer"=w1080, "ToolButtonSelected"=w1079) -> (w1082:refnum<class "Gviewer.lvclass">)
            n457 = Enqueue Element(queue=w1076, element=w1074, error in (no error)=w1078) -> (error out=w1077:errorcluster)  [unwired: 1 in, 2 out]
          }
          frame 5 {
            # "Autoscale Stack"
            n458 = Unbundle By Name(w1089) -> ("YscaleMatch"=w1086:bool, "PrevToolButton"=w1097:i32, "GViewer-Queue"=w1092:refnum<queue>)
            n459 = Get Date/Time In Seconds() -> (seconds since 1Jan1904=w1088:timestamp)
            n460 = Select(t=AutoScale."StackEqual" ("AutoScale"), s=w1086, f=AutoScale."StackMax" ("AutoScale")) -> (s? t:f=w1084:T13)
            n461 = To Variant(anything=w1084) -> (Variant=w1087:variant)
            n462 = To Double Precision Float(number=w1088) -> (double precision float=w1098:dbl)
            n463 = Bundle By Name(cluster=T17 {"ServerActions"=enum."GraphUpdate", "data"=variant, "Source"="", "Time Stamp"=timestamp(0 s since 1904-01-01)} ("element"), "ServerActions"=Typedef_ServerActions."AutoScale", "data"=w1087, "Source"="Toolbar", "Time Stamp"=w1088) -> (w1090:T17)
            n464 = Bundle By Name(cluster=w1089, "AutoScale"=w1084, "AutoscaleContinuous"=FALSE, "ContOnTimer"=w1098, "ToolButtonSelected"=w1097) -> (w1100:refnum<class "Gviewer.lvclass">)
            n465 = Enqueue Element(queue=w1092, element=w1090, error in (no error)=w1094) -> (error out=w1093:errorcluster)  [unwired: 1 in, 2 out]
          }
        }
      }
      event "ToolBar": Mouse Up; "ToolBar": Mouse Leave {
        # "Press a button on the toolbar"
        n466 = event-data() -> ()  [unwired: 1 in, 4 out]
        n467 = call "ToolBarButtonDraw.vi"("error in (no error)"=w1106, "Gviewer in"=w1104) -> ("error out"=w1105:errorcluster, "Gviewer out"=w1102:refnum<class "Gviewer.lvclass">)  [unwired: 8 in]
        n468 = Bundle By Name(cluster=w1102, "ContOnTimer"=-1.0) -> (w1101:refnum<class "Gviewer.lvclass">)
      }
      event Value Change {
        # "Set Graph mode to 'live' (continous updates)"
        n469 = event-data() -> ("NewVal"=w1111:T3)  [unwired: 1 in]
        n470 = Bundle By Name(cluster=w1116, "Live"=w1111) -> (w1110:refnum<class "Gviewer.lvclass">)
        n471 = call "Request_Gserver_Update.vi"("error in (no error)"=w1107, "Gviewer in"=w1110) -> ("error out"=w1112:errorcluster, "Gviewer out"=w1113:refnum<class "Gviewer.lvclass">)  [unwired: 8 in]
        n472 = call "SetGraphTime.vi"("error in (no error)"=w1112, "Gviewer in"=w1113) -> ("error out"=w1114:errorcluster, "Gviewer out"=w1115:refnum<class "Gviewer.lvclass">)  [unwired: 8 in]
        n473 = call "GV_DrawLiveBox.vi"("error in (no error)"=w1114, "Gviewer in"=w1115) -> ("error out"=w1108:errorcluster, "Gviewer out"=w1109:refnum<class "Gviewer.lvclass">)  [unwired: 8 in]
      }
      event Panel Close? {
        # "On closing action of this Graph: Ask the Gserver to perform the closing (to ensure that reference in Gserver is removed)"
        n474 = event-data() -> ()  [unwired: 1 in, 4 out]
        n475 = call "SendDataToServer.vi"("Query_type"=Typedef_QueryType."CloseClient", "Gviewer in"=w1120) -> ("Gviewer out"=w1119:refnum<class "Gviewer.lvclass">)  [unwired: 8 in, 1 out]
        n476 = event-data("Discard?"=TRUE) -> ()  [unwired: 1 in, 1 out]
      }
    }
  }
  n477 = call "GV_Destructor.vi"("error in (no error)"=w10, "Gviewer in"=w1) -> ()  [unwired: 8 in, 2 out]
